vi "EnFlo_Hub.vi"() -> ()   [LabVIEW 2013]
uses:
  Anemometry Sub Vis/Controls/Launch_controls/Open_Calib.ctl
  Anemometry Sub Vis/Controls/Launch_controls/Open_Meas.ctl
  Anemometry Sub Vis/Controls/Launch_controls/Open_Enter_Temp.ctl
  Anemometry Sub Vis/Controls/Launch_controls/Multi_Run_Prog.ctl
  Anemometry Sub Vis/Controls/Launch_controls/EnFlo_arm.ctl
  Anemometry Sub Vis/Controls/Launch_controls/Fast_FID_Valve.ctl
  Anemometry Sub Vis/Controls/Launch_controls/Disp_Setup.ctl
  Anemometry Sub Vis/Controls/Launch_controls/EnFlo_Tun_Setup.ctl
  Anemometry Sub Vis/Controls/Launch_controls/User_Metadata.ctl
  Anemometry Sub Vis/Controls/Launch_controls/Trav_3D_move.ctl
  Anemometry Sub Vis/Controls/Launch_controls/Trav_Space.ctl
  Anemometry Sub Vis/Controls/Launch_controls/Tunnel_speed.ctl
  Anemometry Sub Vis/Controls/Launch_controls/Client_source_control.ctl
  Anemometry Sub Vis/Controls/Launch_controls/Hydrosonic_Manual.ctl
  Anemometry Sub Vis/Controls/Launch_controls/Preference_Panel.ctl
  Anemometry Sub Vis/Controls/Launch_controls/Hot_wire_Calculator.ctl
  Anemometry Sub Vis/Controls/Launch_controls/RW_X_Parker_Config.ctl
  Anemometry Sub Vis/Controls/Launch_controls/LDA_Alignment.ctl
  Anemometry Sub Vis/Controls/Launch_controls/Named_Serial_Comms.ctl
  Anemometry Sub Vis/Controls/Launch_controls/BSA_data_rates.ctl
  Anemometry Sub Vis/Controls/Launch_controls/Serial_Setup.ctl
  Anemometry Sub Vis/Controls/Launch_controls/Post_Process_icon.ctl
  Anemometry Sub Vis/Controls/Launch_controls/Edit_Ascii_file.ctl
  Anemometry Sub Vis/Controls/Launch_controls/Edit_Raw_DF.ctl
  Anemometry Sub Vis/Controls/Launch_controls/Results_file_plotter.ctl
  Anemometry Sub Vis/Controls/Launch_controls/Serial_Port_Names.ctl
  Anemometry Sub Vis/Controls/Launch_controls/Paul.ctl
  Anemometry Sub Vis/Controls/Launch_controls/Tom.ctl
  Anemometry Sub Vis/Controls/Launch_controls/Scani_Valve.ctl
  Anemometry Sub Vis/Controls/Launch_controls/Edit_sever_Channel.ctl
  Anemometry Sub Vis/Controls/Launch_controls/Day_file_plotter.ctl
  Anemometry Sub Vis/Controls/Launch_controls/Plot_Sever_Data.ctl
  Anemometry Sub Vis/Controls/Launch_controls/Adam_Table.ctl
  Anemometry Sub Vis/Controls/Launch_controls/Active_Channel_Control.ctl
  Anemometry Sub Vis/Controls/Setup.ctl
  Anemometry Sub Vis/Controls/Post_Process.ctl
  Anemometry Sub Vis/Controls/Preference_Mode.ctl
  Anemometry Sub Vis/Gen Trav/Trav_mode.ctl
  Anemometry Sub Vis/Controls/User_Specific_mode.ctl
  Anemometry Sub Vis/File/Setup_Filetype.ctl
  Anemometry Sub Vis/Calibration/Calib_mode.ctl
  Anemometry Sub Vis/Controls/Server_Comms.ctl
  Anemometry Sub Vis/Controls/App_Global.ctl
  Anemometry Sub Vis/Globals/Dynamic_call_global.ph.vi
  Anemometry Sub Vis/Globals/Constants_global.vi
  Anemometry Sub Vis/Globals/Preference_global.vi
  Anemometry Sub Vis/Globals/Meas_global.vi
  <vilib>/Platform/browser.llb/Open URL in Default Browser (string).vi
  Anemometry Sub Vis/Globals/Trav_pos_global.vi
  Anemometry Sub Vis/Acquisition/PWA/PWAtasksGLOBAL.vi
  Anemometry Sub Vis/Utilities/Email_transfer_global.vi
panel:
  out "List of ADAM channels to view":string[](array[string])
  out "List of ADAM control channels":string[](array[string])
  out "Analogue Dev Name":string="Dev2"
  out "Numeric":i32
  out "Rig Name":string="EnFlo Tunnel"
  out "All Users":path=path "/System Folder/Preferences/LabVIEW (EnFlo specific)/Meas Setups"
  out "Dummy Measurement":bool
  in  "stop":bool
  in  "Tab Control":T1(tab)
  in  "Tunnel Speed Control":T2
  in  "Traverse Space":T3
  in  "Trav 3D Move":T4 caption="3D Traverse Move"
  in  "User Metadata":T5
  in  "Multi Run Prog":T6
  in  "Enter Temp_Press":T7
  in  "Measurement Prog":T8 caption="Measurement"
  in  "Calibration Prog":T9 caption="Calibration"
  in  "Scani Valve":T10
  in  "LDA Alignment":T11
  in  "Hydrosonic Control":T12
  in  "Fast FID Valve":T13
  in  "Source Control":T14
  in  "Gas Release Setup":T15
  in  "EnFlo Tunnel Setup":T16
  in  "Heater Setup":bool caption="Inlet heater File"
  in  "EnFlo Arm":T17
  in  "EnFlo Tun Display":bool
  in  "Beam Check Positions":bool
  in  "Rig_Control":cluster{"Ch Name":string, "Boolean":bool}[](array[cluster])
  in  "ADAM Channels Control":T18 caption="Change Active Channels"
  in  "ADAM Scan Table":T19 caption="Run ADAM Scan Table"
  in  "Edit Server Channel":T20
  in  "Plot Server Channels":T21 caption="Plot Server Data"
  in  "Day Files Plotter":T22 caption="Plot Data From File"
  out "Current Values":cluster{"Ch Name":string, "Numeric":dbl}[](array[cluster])
  in  "Post_Pro_Results_Hierarchy":bool
  in  "Results File Plotter":T23
  in  "Edit Raw Data Files":T24
  in  "Edit ASCII File":T25
  in  "Post Process Raw Data":T26
  in  "Plot_FFID_Calibs.vi":bool
  in  "Top Level Traverse":bool
  in  "Show Manual Sync":bool
  in  "Sync to server now":bool
  in  "Port Names":T27
  in  "Serial Setup":T28
  in  "LDA Data Rate":T29
  in  "Named Serial Comms":T30
  in  "RW Trav Setup":T31
  in  "Hot Wire Calc":T32
  in  "Preference Panel":T33
  in  "Tom Lawton t.lawton@surrey.ac.uk":T34 caption="For hardware support"
  in  "Paul Hayden p.hayden@surrey.ac.uk":T35 caption="For software support"
  in  "Online Manual":bool
  out "VI Name":string
  out "Iterations":i32
  # "Or give us a call on Tel: 01483 689545"
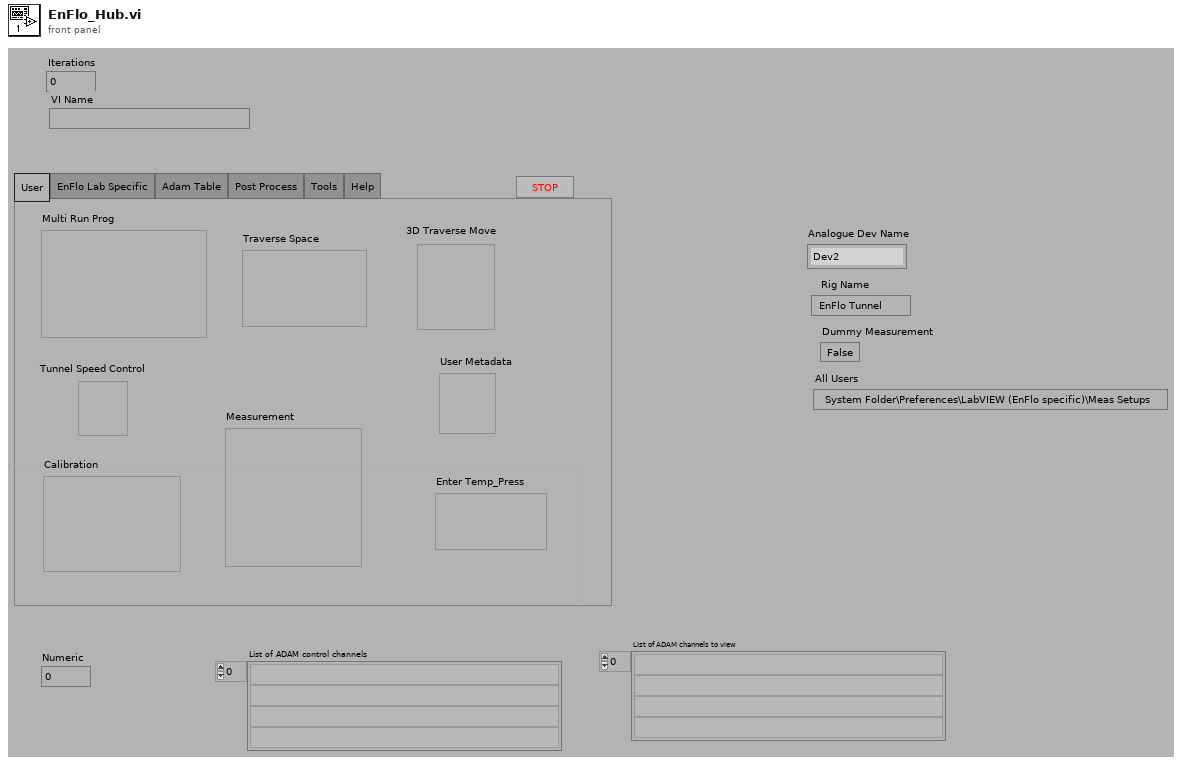
[diagram p1: front panel]
types:
  T1 = enum32{"User", "EnFlo Lab Specific", "Adam Table", "Post Process", "Tools", "Help"}
  T2 = typedef "Tunnel_speed.ctl" = bool
  T3 = typedef "Trav_Space.ctl" = bool
  T4 = typedef "Trav_3D_move.ctl" = bool
  T5 = typedef "User_Metadata.ctl" = bool
  T6 = typedef "Multi_Run_Prog.ctl" = bool
  T7 = typedef "Open_Enter_Temp.ctl" = bool
  T8 = typedef "Open_Meas.ctl" = bool
  T9 = typedef "Open_Calib.ctl" = bool
  T10 = typedef "Scani_Valve.ctl" = bool
  T11 = typedef "LDA_Alignment.ctl" = bool
  T12 = typedef "Hydrosonic_Manual.ctl" = bool
  T13 = typedef "Fast_FID_Valve.ctl" = bool
  T14 = typedef "Client_source_control.ctl" = bool
  T15 = typedef "Disp_Setup.ctl" = bool
  T16 = typedef "EnFlo_Tun_Setup.ctl" = bool
  T17 = typedef "EnFlo_arm.ctl" = bool
  T18 = typedef "Active_Channel_Control.ctl" = bool
  T19 = typedef "Adam_Table.ctl" = bool
  T20 = typedef "Edit_sever_Channel.ctl" = bool
  T21 = typedef "Plot_Sever_Data.ctl" = bool
  T22 = typedef "Day_file_plotter.ctl" = bool
  T23 = typedef "Results_file_plotter.ctl" = bool
  T24 = typedef "Edit_Raw_DF.ctl" = bool
  T25 = typedef "Edit_Ascii_file.ctl" = bool
  T26 = typedef "Post_Process_icon.ctl" = bool
  T27 = typedef "Serial_Port_Names.ctl" = bool
  T28 = typedef "Serial_Setup.ctl" = bool
  T29 = typedef "BSA_data_rates.ctl" = bool
  T30 = typedef "Named_Serial_Comms.ctl" = bool
  T31 = typedef "RW_X_Parker_Config.ctl" = bool
  T32 = typedef "Hot_wire_Calculator.ctl" = bool
  T33 = typedef "Preference_Panel.ctl" = bool
  T34 = typedef "Tom.ctl" = bool
  T35 = typedef "Paul.ctl" = bool
  T36 = typedef "Post_Process.ctl" = enum16{"Take New Data", "Post Process Raw Data File"}
  T37 = typedef "Setup.ctl" = enum16{"Run Program", "Show Setup", "Save Current Setup", "Setup Front Panel"}
  T38 = enum16{"Get Channel Names", "Get Current Value", "Update Channel Value", "Update Channel Description"}
  T39 = enum32{"Invalid", "Standard", "Closed", "Hidden", "Minimized", "Maximized"}
  T40 = enum32{"Bad", "Idle", "Run top level", "Running"}
  T41 = enum16{"Load From Excel File", "Save to Excel File"}
  T42 = typedef "Preference_Mode.ctl" = enum16{"Load Preferences from file", "Save Preferences to file", "Load, Edit then Save"}
  T43 = typedef "User_Specific_mode.ctl" = enum16{"Check VI only", "Run VI"}
  T44 = typedef "Trav_mode.ctl" = enum16{"Move traverse", "Read traverse position", "Teach Position"}
  T45 = typedef "Setup_Filetype.ctl" = enum16{"Measurement Setups", "Calibration Setups", "General", "Results File Plotter Setups", "Speed Calib Tweaks"}
  T46 = enum16{"Load Command File", "Save Command File", "Check Multi Run Prog", "Check Multi Run Prog With Live Moves", "Run Multi Run Prog"}
  T47 = typedef "Calib_mode.ctl" = enum16{"Show Setup", "Take a New Calibration Point", "Refit Curve", "Setup Front Panel"}
  T48 = typedef "Tunnel_Coordinates.ctl" = enum16{"Work in Tunnel Coordinates", "Work in Model Coordinates"}
  T49 = typedef "App_Global.ctl" = enum16{"Read Global", "Write to Global", "Initialise Array"}
  T50 = typedef "App_Ref_Cluster.ctl" = cluster{"Server IP & Port No":string, "Application reference":refnum<vi>}
  T51 = typedef "Server_Comms.ctl" = enum16{"Server Link Healthy", "Do Not Link To Server"}
  T52 = typedef "Ch_description_ADAM.ctl" = cluster{"Ch Name":string, "Type":T53, "Function":T54, "Ch State":T55, "Calibration type":T56, "A":dbl, "B":dbl, "C":dbl, "D":dbl, "Comments":string, "Address":T57, "String":string, "Duty":u16}
  T53 = typedef "Module_type_ADAM.ctl" = string
  T54 = typedef "Function_ADAM.ctl" = enum16{"Analogue Input", "Digital Input", "Event counter", "Event rate", "Analogue Output", "Digital Output", "Relay Output"}
  T55 = typedef "Channel_State.ctl" = enum16{"On", "Off", "Always On", "Always Off"}
  T56 = typedef "Calib_type_ADAM.ctl" = enum16{"Raw", "Bx + A", "Cx^2 + Bx + A", "Dx^3 + Cx^2 + Bx + A", "In Band", "Hi-Tec Q", "Hi-Tec M_dot", "Text"}
  T57 = typedef "Address.ctl" = cluster{"Main":i32, "Ch.":i32, "Sub":i32, "Port Name":string}
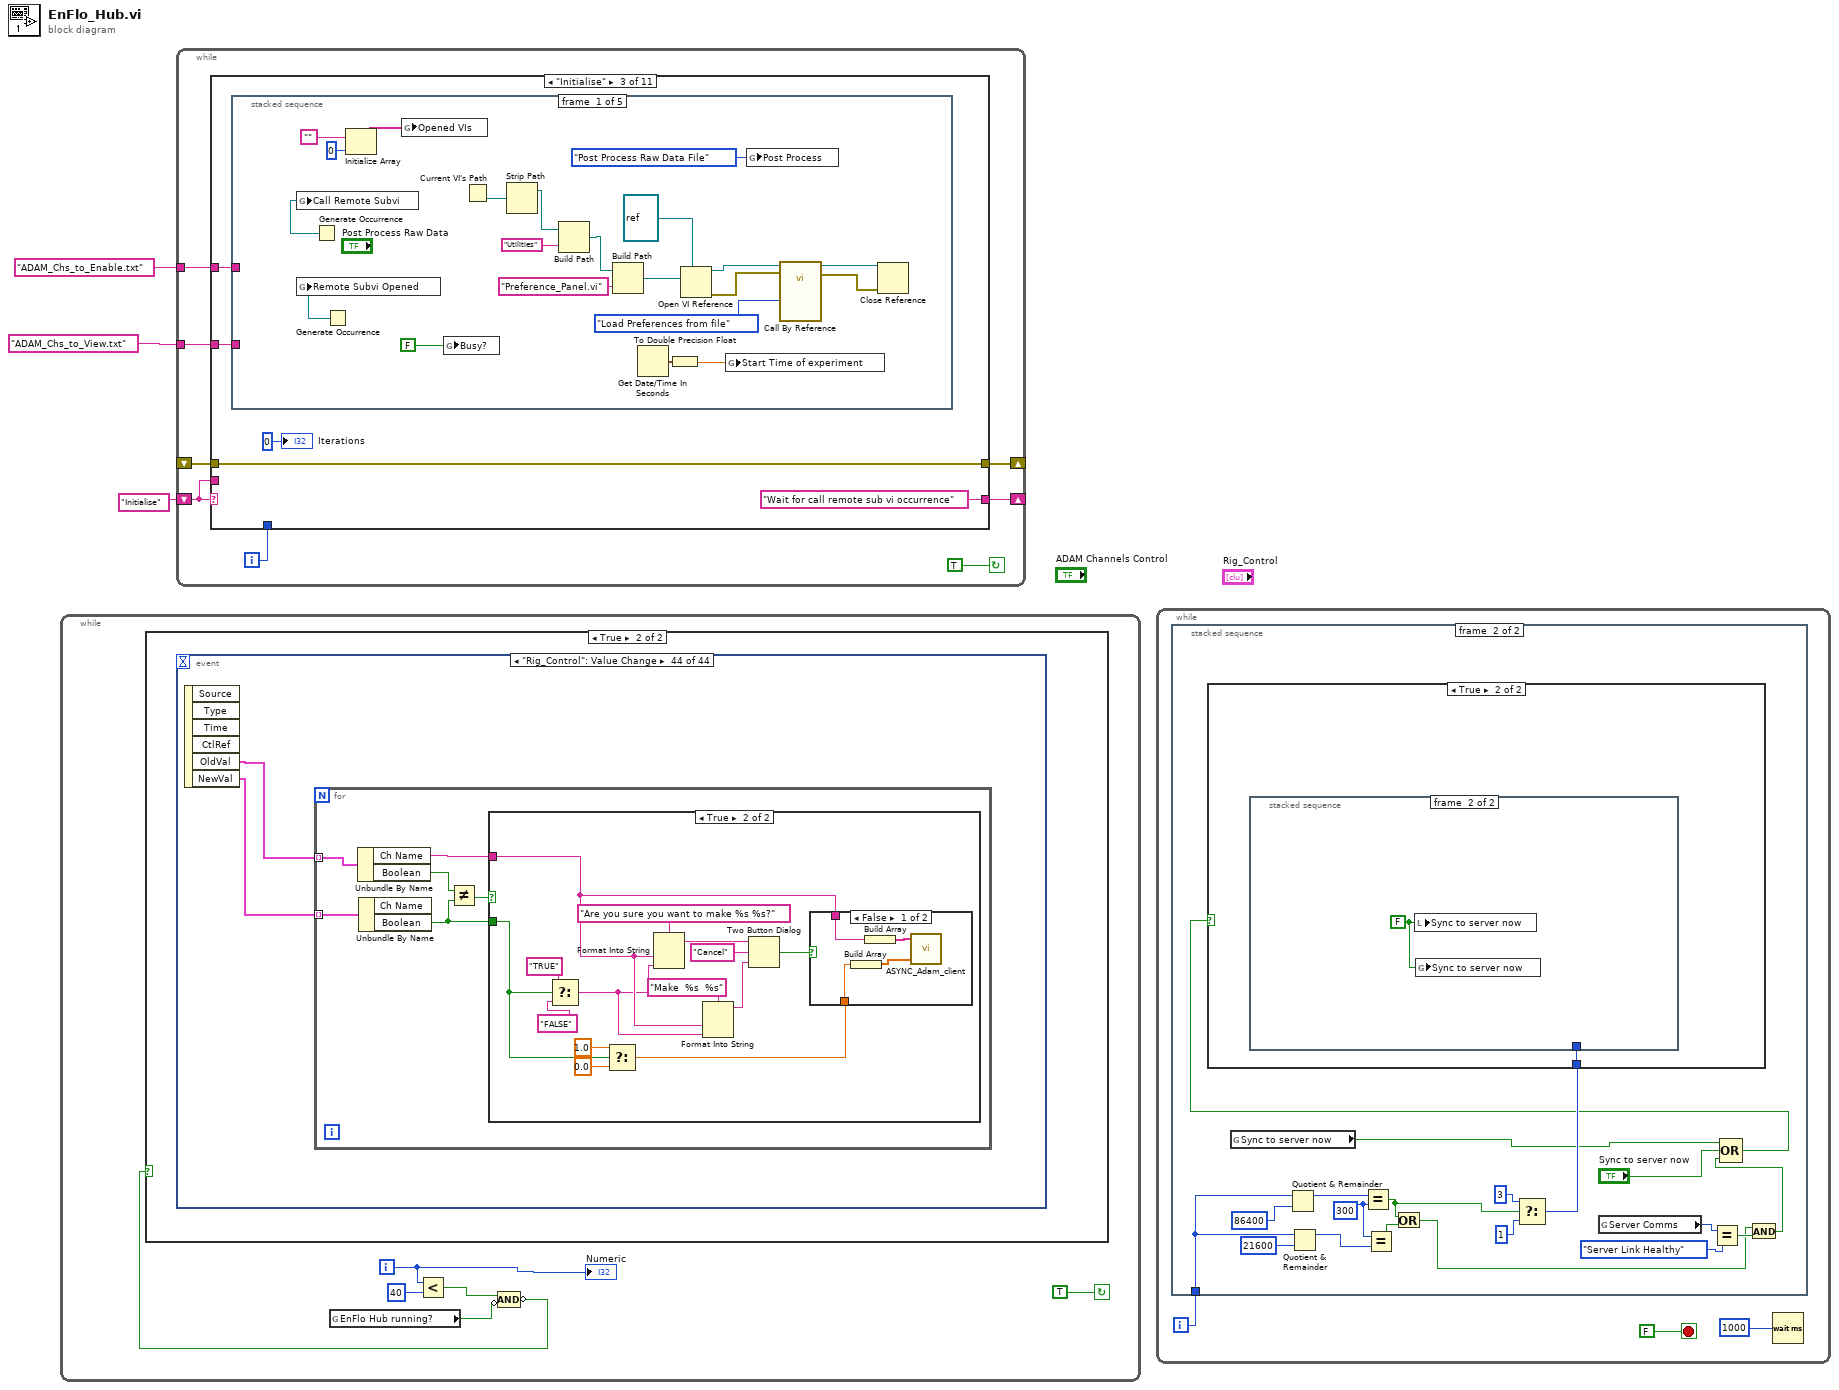
[diagram p0: block diagram]
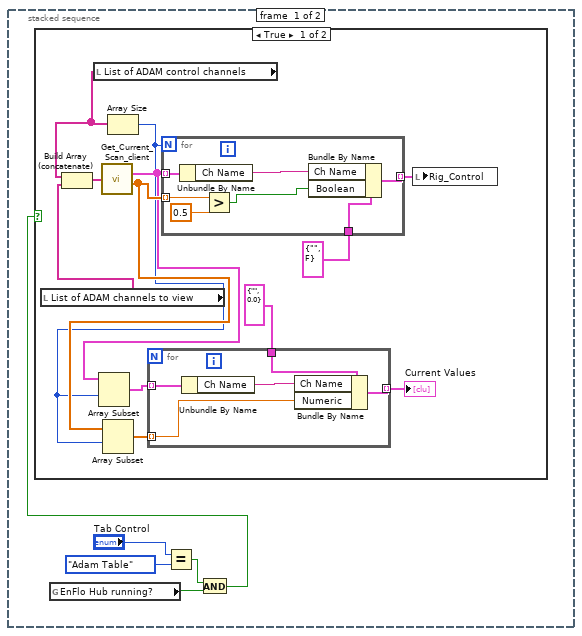
[diagram p2: hidden frame]
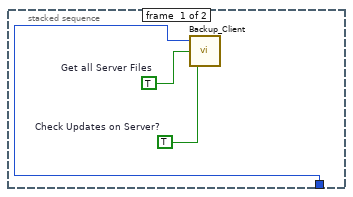
[diagram p5: hidden frame]
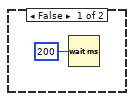
[diagram p6: hidden frame]
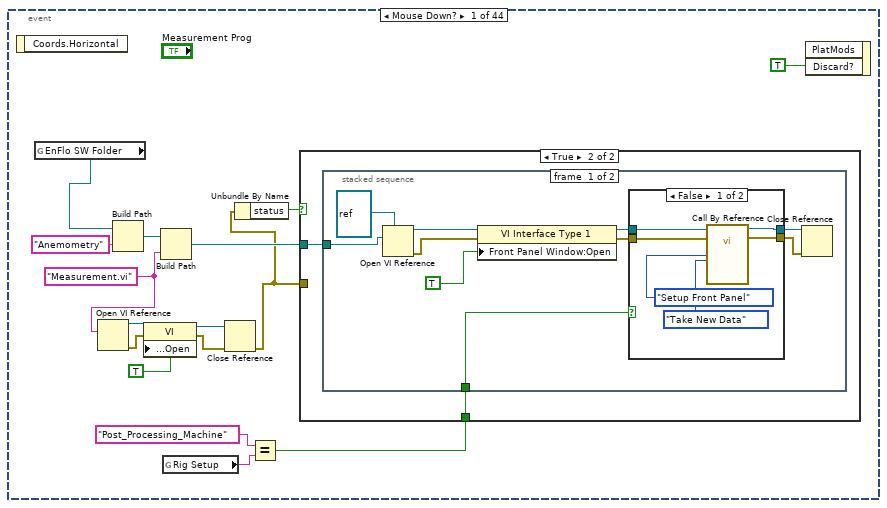
[diagram p7: hidden frame]
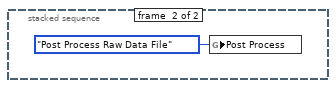
[diagram p10: hidden frame]
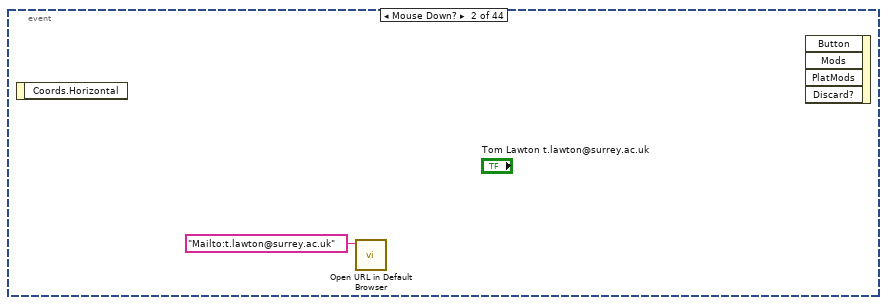
[diagram p11: hidden frame]
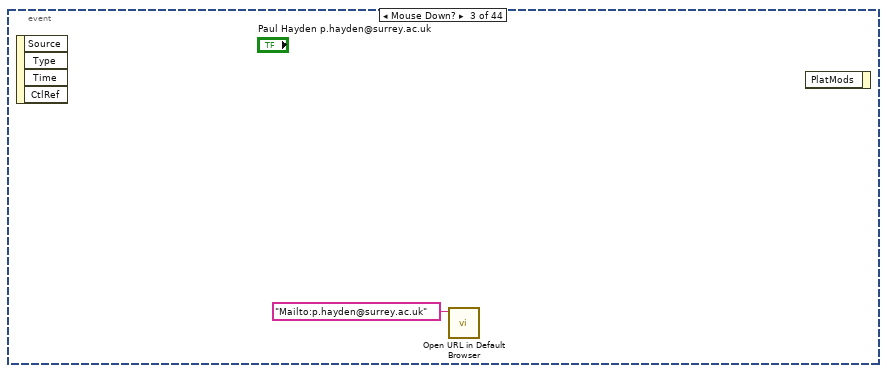
[diagram p12: hidden frame]
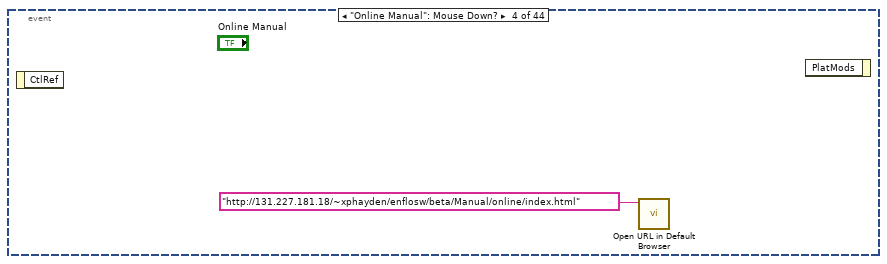
[diagram p13: hidden frame]
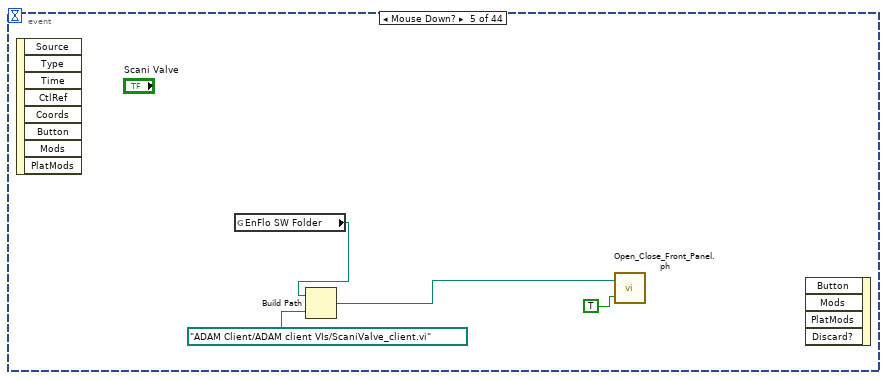
[diagram p14: hidden frame]
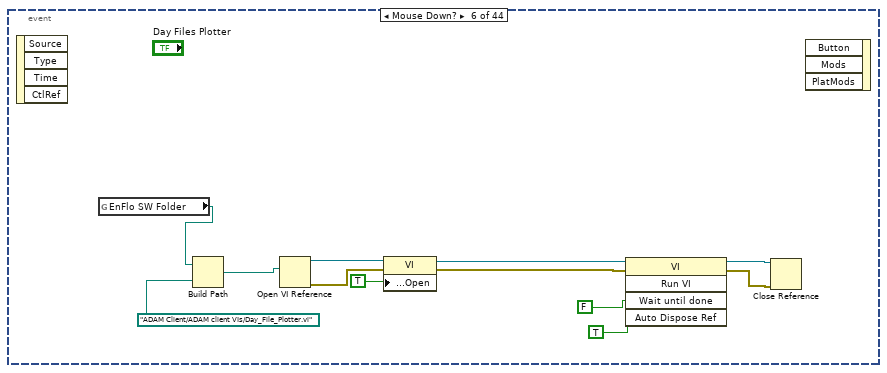
[diagram p15: hidden frame]
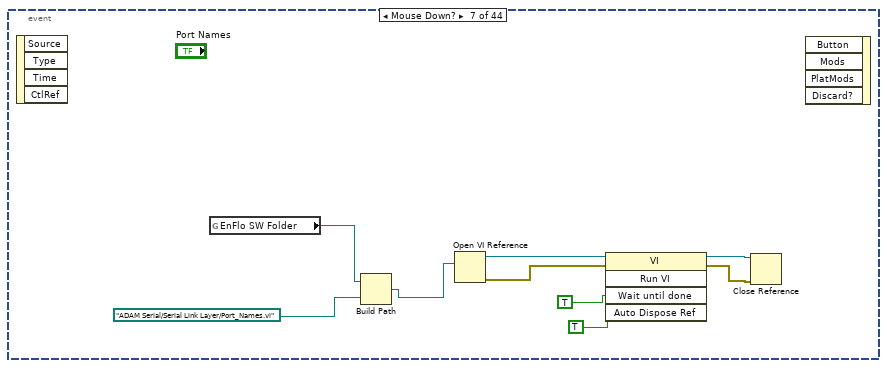
[diagram p16: hidden frame]
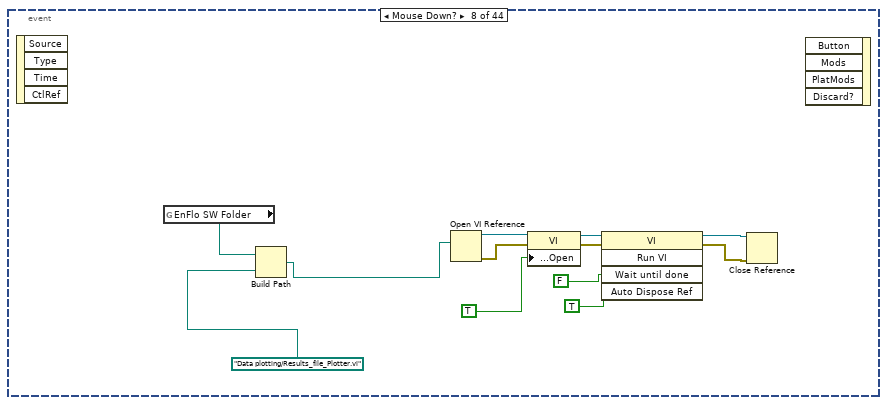
[diagram p17: hidden frame]
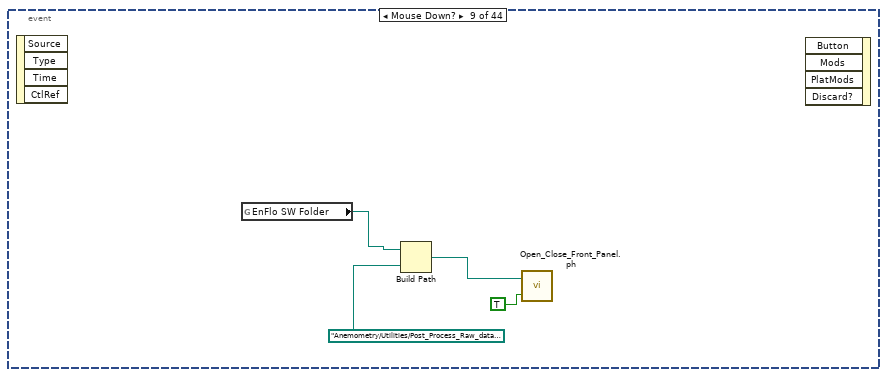
[diagram p18: hidden frame]
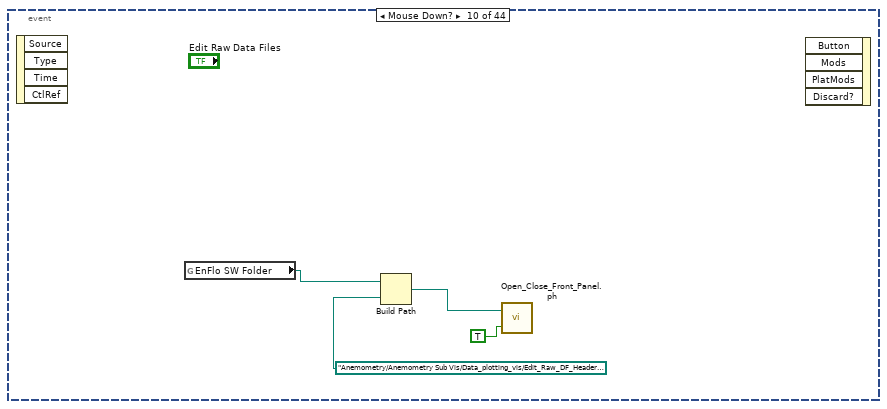
[diagram p19: hidden frame]
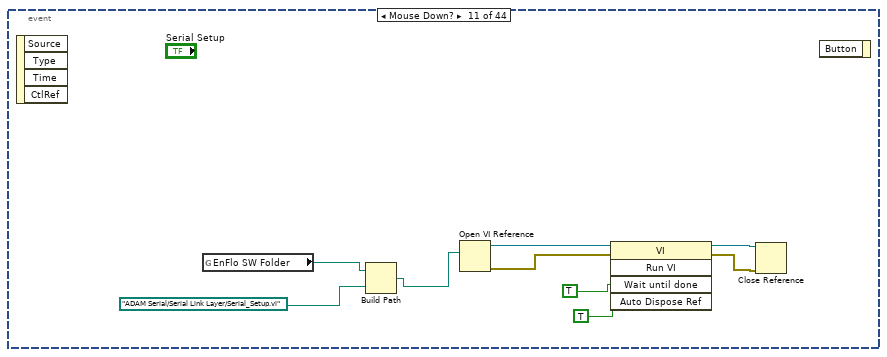
[diagram p20: hidden frame]
diagram:
  n1 = while {
    i -> [w8]
    stop <- TRUE continue-if-true
    n2 = global read "Dynamic_call_global.ph.vi" "EnFlo Hub running?"() -> (w6:bool)
    n3 = Less?(x=w8, y=40) -> (x < y?=w5:bool)
    n4 = Compound Arithmetic op=AND(w5, invert w6) -> (invert w4:bool)
    n5 = case shown="True" w4 {
      frame False {
        n6 = Wait (ms)(milliseconds to wait=u32 200) -> ()  [unwired: 1 out]
      }
      frame True {
        n7 = event shown="[43] \"Rig_Control\": Value Change" {
          selector: _ -> [_ _ _ _ _ _ _ _ _ _ _ _ _ _ _ _ _ _ _ _ _ _ _ _ _ _ _ _ _ _ _ _ _ _ _ _ _ _ _ _ _ _ _ _]
          dyn-events: _ -> [_ _ _ _ _ _ _ _ _ _ _ _ _ _ _ _ _ _ _ _ _ _ _ _ _ _ _ _ _ _ _ _ _ _ _ _ _ _ _ _ _ _ _ _]
          timeout: _ -> [_ _ _ _ _ _ _ _ _ _ _ _ _ _ _ _ _ _ _ _ _ _ _ _ _ _ _ _ _ _ _ _ _ _ _ _ _ _ _ _ _ _ _ _]
          event Mouse Down? {
            w19 = "Measurement.vi" ("name or relative path")
            n8 = event-data() -> ()  [unwired: 2 out]
            n9 = global read "Constants_global.vi" "EnFlo SW Folder"() -> (w22:path)
            n10 = Open VI Reference(vi path=w19) -> (vi reference=w18:refnum<vi>, error out=w17:errorcluster)  [unwired: 1 in, 4 out]
            n11 = Build Path(base path=w22, name or relative path="Anemometry") -> (appended path=w25:path)
            n12 = property class="VI"(reference=w18, error in=w17, "Front Panel Window:Open"=TRUE) -> (reference out=w15:refnum<vi>, error out=w16:errorcluster)
            n13 = Build Path(base path=w25, name or relative path=w19) -> (appended path=w23:path)
            n14 = global read "Preference_global.vi" "Rig Setup"() -> (w13:string)
            n15 = Close Reference(reference=w15, error in (no error)=w16) -> (error out=w14:errorcluster)
            n16 = Unbundle By Name(w14) -> ("status"=w24:bool)
            n17 = Equal?(x="Post_Processing_Machine" ("Rig Setup"), y=w13) -> (x = y?=w11:bool)
            n18 = case shown="True" w24 {
              tunnel: w23 -> [_ w28]
              tunnel: w14 -> [_ _]
              tunnel: w11 -> [_ w27]
              frame False {
              }
              frame True {
                n19 = stacked-sequence {
                  tunnel: w28 -> [w38 _]
                  tunnel: w27 -> [w29 _]
                  frame #0 {
                    n20 = Open VI Reference(type specifier VI Refnum (for type only)=refnum<vi> refnum, vi path=w38) -> (vi reference=w36:refnum<vi>, error out=w35:errorcluster)  [unwired: 1 in, 3 out]
                    n21 = property class="VI Interface Type 1"(reference=w36, error in=w35, "Front Panel Window:Open"=TRUE) -> (reference out=w31:refnum<vi>, error out=w30:errorcluster)
                    n22 = case shown="False" w29 {
                      tunnel: [w44 w46] -> w34
                      tunnel: [w43 w45] -> w33
                      tunnel: w31 -> [w42 w46]
                      tunnel: w30 -> [w41 w45]
                      frame False {
                        n23 = call-by-ref "?"(reference=w42, error in=w41, "setup"=Setup."Setup Front Panel", "Post Process"=Post_Process."Take New Data") -> (reference out=w44:refnum<vi>, error out=w43:errorcluster)  [unwired: 16 in, 2 out]
                      }
                      frame True {
                      }
                    }
                    n24 = Close Reference(reference=w34, error in (no error)=w33) -> ()  [unwired: 1 out]
                  }
                  frame #1 {
                    n25 = global write "Meas_global.vi" "Post Process"(Post_Process."Post Process Raw Data File" ("Post Process")) -> ()
                  }
                }
              }
            }
            n26 = event-data("Discard?"=TRUE) -> ()  [unwired: 1 in, 2 out]
          }
          event Mouse Down? {
            n27 = event-data() -> ()  [unwired: 2 out]
            n28 = call-poly <vilib>:"Open URL in Default Browser.vi"("URL"="Mailto:t.lawton@surrey.ac.uk") -> ()  [unwired: 1 in, 6 out]
            n29 = event-data() -> ()  [unwired: 1 in, 5 out]
          }
          event Mouse Down? {
            n30 = event-data() -> ()  [unwired: 5 out]
            n31 = call-poly <vilib>:"Open URL in Default Browser.vi"("URL"="Mailto:p.hayden@surrey.ac.uk") -> ()  [unwired: 1 in, 6 out]
            n32 = event-data() -> ()  [unwired: 1 in, 2 out]
          }
          event "Online Manual": Mouse Down? {
            n33 = event-data() -> ()  [unwired: 2 out]
            n34 = call-poly <vilib>:"Open URL in Default Browser.vi"("URL"="http://131.227.181.18/~xphayden/enflosw/beta/Manual/online/index.html") -> ()  [unwired: 1 in, 6 out]
            n35 = event-data() -> ()  [unwired: 1 in, 2 out]
          }
          event Mouse Down? {
            n36 = event-data() -> ()  [unwired: 9 out]
            n37 = global read "Constants_global.vi" "EnFlo SW Folder"() -> (w51:path)
            n38 = Build Path(base path=w51, name or relative path=path "ADAM Client/ADAM client VIs/ScaniValve_client.vi") -> (appended path=w54:path)
            n39 = call "Open_Close_Front_Panel.ph.vi"("Front Panel Window:Open"=TRUE, "VI path"=w54) -> ()  [unwired: 2 out]
            n40 = event-data() -> ()  [unwired: 1 in, 5 out]
          }
          event Mouse Down? {
            n41 = event-data() -> ()  [unwired: 5 out]
            n42 = global read "Constants_global.vi" "EnFlo SW Folder"() -> (w55:path)
            n43 = Build Path(base path=w55, name or relative path=path "ADAM Client/ADAM client VIs/Day_File_Plotter.vi") -> (appended path=w61:path)
            n44 = Open VI Reference(vi path=w61) -> (vi reference=w62:refnum<vi>, error out=w64:errorcluster)  [unwired: 2 in, 3 out]
            n45 = property class="VI"(reference=w62, error in=w64, "Front Panel Window:Open"=TRUE) -> (reference out=w66:refnum<vi>, error out=w65:errorcluster)
            n46 = invoke class="VI" method="Run VI"(reference=w66, error in=w65, "Wait until done"=FALSE, "Auto Dispose Ref"=TRUE) -> (reference out=w57:refnum<vi>, error out=w58:errorcluster)  [unwired: 1 in, 3 out]
            n47 = Close Reference(reference=w57, error in (no error)=w58) -> ()  [unwired: 1 out]
            n48 = event-data() -> ()  [unwired: 1 in, 4 out]
          }
          event Mouse Down? {
            n49 = event-data() -> ()  [unwired: 5 out]
            n50 = global read "Constants_global.vi" "EnFlo SW Folder"() -> (w67:path)
            n51 = Build Path(base path=w67, name or relative path=path "ADAM Serial/Serial Link Layer/Port_Names.vi") -> (appended path=w69:path)
            n52 = Open VI Reference(vi path=w69) -> (vi reference=w74:refnum<vi>, error out=w75:errorcluster)  [unwired: 1 in, 4 out]
            n53 = invoke class="VI" method="Run VI"(reference=w74, error in=w75, "Wait until done"=TRUE, "Auto Dispose Ref"=TRUE) -> (reference out=w70:refnum<vi>, error out=w71:errorcluster)  [unwired: 1 in, 3 out]
            n54 = Close Reference(reference=w70, error in (no error)=w71) -> ()  [unwired: 1 out]
            n55 = event-data() -> ()  [unwired: 1 in, 5 out]
          }
          event Mouse Down? {
            n56 = event-data() -> ()  [unwired: 5 out]
            n57 = global read "Constants_global.vi" "EnFlo SW Folder"() -> (w76:path)
            n58 = Build Path(base path=w76, name or relative path=path "Data plotting/Results_file_Plotter.vi") -> (appended path=w79:path)
            n59 = Open VI Reference(vi path=w79) -> (vi reference=w81:refnum<vi>, error out=w78:errorcluster)  [unwired: 1 in, 4 out]
            n60 = property class="VI"(reference=w81, error in=w78, "Front Panel Window:Open"=TRUE) -> (reference out=w82:refnum<vi>, error out=w83:errorcluster)
            n61 = invoke class="VI" method="Run VI"(reference=w82, error in=w83, "Wait until done"=FALSE, "Auto Dispose Ref"=TRUE) -> (reference out=w84:refnum<vi>, error out=w85:errorcluster)  [unwired: 1 in, 3 out]
            n62 = Close Reference(reference=w84, error in (no error)=w85) -> ()  [unwired: 1 out]
            n63 = event-data() -> ()  [unwired: 1 in, 5 out]
          }
          event Mouse Down? {
            n64 = event-data() -> ()  [unwired: 5 out]
            n65 = global read "Constants_global.vi" "EnFlo SW Folder"() -> (w88:path)
            n66 = Build Path(base path=w88, name or relative path=path "Anemometry/Utilities/Post_Process_Raw_data.vi") -> (appended path=w90:path)
            n67 = call "Open_Close_Front_Panel.ph.vi"("Front Panel Window:Open"=TRUE, "VI path"=w90) -> ()  [unwired: 2 out]
            n68 = event-data() -> ()  [unwired: 1 in, 5 out]
          }
          event Mouse Down? {
            n69 = event-data() -> ()  [unwired: 5 out]
            n70 = global read "Constants_global.vi" "EnFlo SW Folder"() -> (w92:path)
            n71 = Build Path(base path=w92, name or relative path=path "Anemometry/Anemometry Sub Vis/Data_plotting_vis/Edit_Raw_DF_Header.vi") -> (appended path=w94:path)
            n72 = call "Open_Close_Front_Panel.ph.vi"("Front Panel Window:Open"=TRUE, "VI path"=w94) -> ()  [unwired: 2 out]
            n73 = event-data() -> ()  [unwired: 1 in, 5 out]
          }
          event Mouse Down? {
            n74 = event-data() -> ()  [unwired: 5 out]
            n75 = global read "Constants_global.vi" "EnFlo SW Folder"() -> (w96:path)
            n76 = Build Path(base path=w96, name or relative path=path "ADAM Serial/Serial Link Layer/Serial_Setup.vi") -> (appended path=w98:path)
            n77 = Open VI Reference(vi path=w98) -> (vi reference=w103:refnum<vi>, error out=w104:errorcluster)  [unwired: 1 in, 4 out]
            n78 = invoke class="VI" method="Run VI"(reference=w103, error in=w104, "Wait until done"=TRUE, "Auto Dispose Ref"=TRUE) -> (reference out=w99:refnum<vi>, error out=w100:errorcluster)  [unwired: 1 in, 3 out]
            n79 = Close Reference(reference=w99, error in (no error)=w100) -> ()  [unwired: 1 out]
            n80 = event-data() -> ()  [unwired: 1 in, 2 out]
          }
          event Mouse Down? {
            n81 = event-data() -> ()  [unwired: 5 out]
            n82 = global read "Constants_global.vi" "EnFlo SW Folder"() -> (w106:path)
            n83 = Build Path(base path=w106, name or relative path=path "ADAM Serial/Serial Link Layer/Named_Serial_Comms.vi") -> (appended path=w108:path)
            n84 = call "Open_Close_Front_Panel.ph.vi"("Front Panel Window:Open"=TRUE, "VI path"=w108) -> ()  [unwired: 2 out]
            n85 = event-data() -> ()  [unwired: 1 in, 5 out]
          }
          event Mouse Down? {
            n86 = event-data() -> ()  [unwired: 5 out]
            n87 = global read "Constants_global.vi" "EnFlo SW Folder"() -> (w109:path)
            n88 = Build Path(base path=w109, name or relative path=path "Anemometry/Anemometry Sub Vis/LDA/LDA_data_rate.vi") -> (appended path=w111:path)
            n89 = call "Open_Close_Front_Panel.ph.vi"("Front Panel Window:Open"=TRUE, "VI path"=w111) -> ()  [unwired: 2 out]
            n90 = event-data() -> ()  [unwired: 1 in, 2 out]
          }
          event Mouse Down? {
            n91 = event-data() -> ()  [unwired: 5 out]
            n92 = global read "Constants_global.vi" "EnFlo SW Folder"() -> (w123:path)
            n93 = Build Path(base path=w123, name or relative path=path "ADAM Client/ADAM client VIs/Control_Channel_Status.vi") -> (appended path=w113:path)
            n94 = Open VI Reference(vi path=w113) -> (vi reference=w116:refnum<vi>, error out=w114:errorcluster)  [unwired: 1 in, 4 out]
            n95 = property class="VI"(reference=w116, error in=w114, "Front Panel Window:Open"=TRUE) -> (reference out=w117:refnum<vi>, error out=w118:errorcluster)
            n96 = invoke class="VI" method="Run VI"(reference=w117, error in=w118, "Wait until done"=FALSE, "Auto Dispose Ref"=TRUE) -> (reference out=w119:refnum<vi>, error out=w120:errorcluster)  [unwired: 1 in, 3 out]
            n97 = Close Reference(reference=w119, error in (no error)=w120) -> ()  [unwired: 1 out]
            n98 = event-data() -> ()  [unwired: 1 in, 2 out]
          }
          event Mouse Down? {
            n99 = event-data() -> ()  [unwired: 5 out]
            n100 = global read "Constants_global.vi" "EnFlo SW Folder"() -> (w125:path)
            n101 = Build Path(base path=w125, name or relative path=path "Anemometry/Utilities/LDA_Beam_Alignment.vi") -> (appended path=w127:path)
            n102 = call "Open_Close_Front_Panel.ph.vi"("Front Panel Window:Open"=TRUE, "VI path"=w127) -> ()  [unwired: 2 out]
            n103 = event-data() -> ()  [unwired: 1 in, 5 out]
          }
          event Mouse Down? {
            w130 = FALSE  # Wait until done
            n104 = event-data() -> ()  [unwired: 5 out]
            n105 = call "Run_Enter_Temp.vi"("Wait until done"=w130) -> ()  [unwired: 1 out]
            n106 = event-data("Discard?"=TRUE) -> ()  [unwired: 1 in, 4 out]
          }
          event Mouse Down? {
            n107 = event-data() -> ()  [unwired: 5 out]
            n108 = global read "Constants_global.vi" "EnFlo SW Folder"() -> (w131:path)
            n109 = Build Path(base path=w131, name or relative path=path "Anemometry/Utilities/Edit_ASCI_file.vi") -> (appended path=w134:path)
            n110 = call "Open_Close_Front_Panel.ph.vi"("Front Panel Window:Open"=TRUE, "VI path"=w134) -> ()  [unwired: 2 out]
            n111 = event-data() -> ()  [unwired: 1 in, 5 out]
          }
          event "Heater Setup": Mouse Down? {
            n112 = event-data() -> ()  [unwired: 5 out]
            n113 = global read "Constants_global.vi" "EnFlo SW Folder"() -> (w135:path)
            n114 = Build Path(base path=w135, name or relative path=path "Anemometry/Utilities/Create_Heater_Setpoints_File.vi") -> (appended path=w138:path)
            n115 = call "Open_Close_Front_Panel.ph.vi"("Front Panel Window:Open"=TRUE, "VI path"=w138) -> ()  [unwired: 2 out]
            n116 = event-data() -> ()  [unwired: 1 in, 5 out]
          }
          event Mouse Down? {
            n117 = event-data() -> ()  [unwired: 5 out]
            n118 = global read "Constants_global.vi" "EnFlo SW Folder"() -> (w139:path)
            n119 = Build Path(base path=w139, name or relative path=path "ADAM Client/Sub VIs/Gas_Release_Control.vi") -> (appended path=w142:path)
            n120 = call "Open_Close_Front_Panel.ph.vi"("Front Panel Window:Open"=TRUE, "VI path"=w142) -> ()  [unwired: 2 out]
            n121 = event-data() -> ()  [unwired: 1 in, 5 out]
          }
          event Mouse Down? {
            n122 = event-data() -> ()  [unwired: 5 out]
            n123 = global read "Constants_global.vi" "EnFlo SW Folder"() -> (w143:path)
            n124 = Build Path(base path=w143, name or relative path=path "ADAM Client/ADAM client VIs/Edit_Server_Channel.vi") -> (appended path=w153:path)
            n125 = Open VI Reference(type specifier VI Refnum (for type only)=refnum<vi> refnum, vi path=w153) -> (vi reference=w146:refnum<vi>, error out=w147:errorcluster)  [unwired: 1 in, 3 out]
            n126 = property class="VI Interface Type 2"(reference=w146, error in=w147, "Front Panel Window:Open"=TRUE) -> (reference out=w149:refnum<vi>, error out=w150:errorcluster)
            n127 = call-by-ref "?"(reference=w149, error in=w150, "Mode"=T38."Get Channel Names") -> (reference out=w151:refnum<vi>, error out=w152:errorcluster)  [unwired: 5 in]
            n128 = Close Reference(reference=w151, error in (no error)=w152) -> ()  [unwired: 1 out]
            n129 = event-data() -> ()  [unwired: 1 in, 5 out]
          }
          event "EnFlo Tun Display": Mouse Down? {
            n130 = event-data() -> ()  [unwired: 9 out]
            n131 = global read "Constants_global.vi" "EnFlo SW Folder"() -> (w166:path)
            n132 = Build Path(base path=w166, name or relative path=path "Anemometry/Utilities/EnFlo_Tunnel_Display.vi") -> (appended path=w161:path)
            n133 = Open VI Reference(vi path=w161) -> (vi reference=w160:refnum<vi>, error out=w159:errorcluster)  [unwired: 5 in]
            n134 = invoke class="VI" method="FP.Open"(reference=w160, error in=w159, "Activate"=TRUE ("Activate?"), "State"=T39."Standard") -> (reference out=w158:refnum<vi>, error out=w157:errorcluster)  [unwired: 1 in, 3 out]
            n135 = invoke class="VI" method="Run VI"(reference=w158, error in=w157, "Wait until done"=FALSE ("Wait Until Done"), "Auto Dispose Ref"=FALSE ("Wait until done")) -> (reference out=w162:refnum<vi>, error out=w163:errorcluster)  [unwired: 1 in, 3 out]
            n136 = Close Reference(reference=w162, error in (no error)=w163) -> ()  [unwired: 1 out]
            n137 = event-data() -> ()  [unwired: 5 in, 1 out]
          }
          event Mouse Down? {
            n138 = event-data() -> ()  [unwired: 5 out]
            n139 = global read "Constants_global.vi" "EnFlo SW Folder"() -> (w168:path)
            n140 = Build Path(base path=w168, name or relative path=path "ADAM Client/ADAM client VIs/Set_Tunnel_Speed.vi") -> (appended path=w171:path)
            n141 = call "Open_Close_Front_Panel.ph.vi"("Front Panel Window:Open"=TRUE, "VI path"=w171) -> ()  [unwired: 2 out]
            n142 = event-data() -> ()  [unwired: 1 in, 5 out]
          }
          event Mouse Down? {
            n143 = event-data() -> ()  [unwired: 5 out]
            n144 = global read "Constants_global.vi" "EnFlo SW Folder"() -> (w172:path)
            n145 = Build Path(base path=w172, name or relative path=path "ADAM Client/ADAM client VIs/Plot_Server_Data.vi") -> (appended path=w175:path)
            n146 = Open VI Reference(vi path=w175) -> (vi reference=w177:refnum<vi>, error out=w174:errorcluster)  [unwired: 1 in, 4 out]
            n147 = property class="VI"(reference=w177, error in=w174, "Front Panel Window:Open"=TRUE) -> (reference out=w178:refnum<vi>, error out=w179:errorcluster)
            n148 = invoke class="VI" method="Run VI"(reference=w178, error in=w179, "Wait until done"=FALSE, "Auto Dispose Ref"=TRUE) -> (reference out=w180:refnum<vi>, error out=w181:errorcluster)  [unwired: 1 in, 3 out]
            n149 = Close Reference(reference=w180, error in (no error)=w181) -> ()  [unwired: 1 out]
            n150 = event-data() -> ()  [unwired: 1 in, 5 out]
          }
          event Mouse Down? {
            n151 = event-data() -> ()  [unwired: 5 out]
            n152 = global read "Constants_global.vi" "EnFlo SW Folder"() -> (w191:path)
            n153 = Build Path(base path=w191, name or relative path=path "ADAM Server/ADAM_scan_table.vi") -> (appended path=w189:path)
            n154 = Open VI Reference(vi path=w189) -> (vi reference=w192:refnum<vi>, error out=w193:errorcluster)  [unwired: 1 in, 4 out]
            n155 = property class="VI"(reference=w192, error in=w193) -> (reference out=w187:refnum<vi>, error out=w186:errorcluster, "Execution:State"=w194:T40)
            n156 = Equal?(x=w194, y=T40."Run top level" ("Execution:State")) -> (x = y?=w188:bool)
            n157 = case shown="False" w188 {
              tunnel: w187 -> [w199 w216]
              tunnel: w186 -> [w198 w215]
              tunnel: [w197 w216] -> w185
              tunnel: [w196 w215] -> w184
              frame False {
                n158 = Two Button Dialog(message="Are you sure that you want to Run the ADAM Scan table on this machine?", 1:"Run" ("F button name (\"Cancel\")"), 2:"Cancel" ("T button name (\"OK\")")) -> (T button?=w200:bool)
                n159 = case shown="False" w200 {
                  tunnel: w199 -> [w207 w214]
                  tunnel: w198 -> [w206 w213]
                  tunnel: [w205 w214] -> w197
                  tunnel: [w204 w213] -> w196
                  frame False {
                    n160 = property class="VI"(reference=w207, error in=w206, "Front Panel Window:Open"=TRUE) -> (reference out=w211:refnum<vi>, error out=w210:errorcluster)
                    n161 = invoke class="VI" method="Run VI"(reference=w211, error in=w210, "Wait until done"=FALSE, "Auto Dispose Ref"=TRUE) -> (reference out=w205:refnum<vi>, error out=w204:errorcluster)  [unwired: 1 in, 3 out]
                  }
                  frame True {
                  }
                }
              }
              frame True {
              }
            }
            n162 = event-data() -> ()  [unwired: 1 in, 2 out]
            n163 = Close Reference(reference=w185, error in (no error)=w184) -> ()  [unwired: 1 out]
          }
          event Mouse Down? {
            n164 = event-data() -> ()  [unwired: 5 out]
            n165 = global read "Constants_global.vi" "EnFlo SW Folder"() -> (w219:path)
            n166 = Build Path(base path=w219, name or relative path=path "ADAM Serial/Instrument drivers/Traverses/~subVIs/Read_Write_Trav_Config.vi") -> (appended path=w220:path)
            n167 = Build Path(base path=w219, name or relative path=path "ADAM Serial/Instrument drivers/Traverses/~subVIs/DriveConfigGlobal.vi") -> (appended path=w221:path)
            n168 = flat-sequence {
              tunnel: w221 -> [w222]
              tunnel: w220 -> [w224]
              frame #0 {
                n169 = call "Open_Close_Front_Panel.ph.vi"("Front Panel Window:Open"=TRUE, "VI path"=w222) -> ()  [unwired: 2 out]
              }
              frame #1 {
                n170 = call "Open_Close_Front_Panel.ph.vi"("Front Panel Window:Open"=TRUE, "VI path"=w224) -> ()  [unwired: 2 out]
              }
            }
            n171 = event-data() -> ()  [unwired: 1 in, 5 out]
          }
          event Mouse Down? {
            n172 = event-data() -> ()  [unwired: 5 out]
            n173 = global read "Constants_global.vi" "EnFlo SW Folder"() -> (w226:path)
            n174 = Build Path(base path=w226, name or relative path=path "Anemometry/Utilities/Hot_wire_Calculator.vi") -> (appended path=w229:path)
            n175 = call "Open_Close_Front_Panel.ph.vi"("Front Panel Window:Open"=TRUE, "VI path"=w229) -> ()  [unwired: 2 out]
            n176 = event-data() -> ()  [unwired: 1 in, 5 out]
          }
          event "Show Manual Sync": Mouse Down {
            n177 = event-data() -> ()  [unwired: 9 out]
            n178 = global read "Constants_global.vi" "EnFlo SW Folder"() -> (w230:path)
            n179 = Build Path(base path=w230, name or relative path=path "Anemometry/Utilities/EnFlo_Data_Sync_Manual.vi") -> (appended path=w233:path)
            n180 = call "Open_Close_Front_Panel.ph.vi"("Front Panel Window:Open"=TRUE, "VI path"=w233) -> ()  [unwired: 2 out]
          }
          event "Plot_FFID_Calibs.vi": Mouse Down {
            n181 = event-data() -> ()  [unwired: 9 out]
            n182 = global read "Constants_global.vi" "EnFlo SW Folder"() -> (w244:path)
            n183 = Build Path(base path=w244, name or relative path=path "ADAM Client/ADAM client VIs/Plot_FFID_Calibs.vi") -> (appended path=w234:path)
            n184 = Open VI Reference(vi path=w234) -> (vi reference=w237:refnum<vi>, error out=w235:errorcluster)  [unwired: 1 in, 4 out]
            n185 = property class="VI"(reference=w237, error in=w235, "Front Panel Window:Open"=TRUE) -> (reference out=w238:refnum<vi>, error out=w239:errorcluster)
            n186 = invoke class="VI" method="Run VI"(reference=w238, error in=w239, "Wait until done"=FALSE, "Auto Dispose Ref"=TRUE) -> (reference out=w240:refnum<vi>, error out=w241:errorcluster)  [unwired: 1 in, 3 out]
            n187 = Close Reference(reference=w240, error in (no error)=w241) -> ()  [unwired: 1 out]
          }
          event "Beam Check Positions": Mouse Down {
            n188 = event-data() -> ()  [unwired: 9 out]
            n189 = global read "Constants_global.vi" "EnFlo SW Folder"() -> (w256:path)
            n190 = Build Path(base path=w256, name or relative path=path "Anemometry/Anemometry Sub Vis/LDA/Beam_Check_Positions.vi") -> (appended path=w247:path)
            n191 = Open VI Reference(type specifier VI Refnum (for type only)=refnum<vi> refnum, vi path=w247) -> (vi reference=w249:refnum<vi>, error out=w250:errorcluster)  [unwired: 1 in, 3 out]
            n192 = property class="VI Interface Type 3"(reference=w249, error in=w250, "Front Panel Window:Open"=TRUE) -> (reference out=w252:refnum<vi>, error out=w253:errorcluster)
            n193 = call-by-ref "?"(reference=w252, error in=w253, "Mode"=T41."Load From Excel File") -> (reference out=w254:refnum<vi>, error out=w255:errorcluster)  [unwired: 2 in, 1 out]
            n194 = Close Reference(reference=w254, error in (no error)=w255) -> ()  [unwired: 1 out]
          }
          event Mouse Down? {
            n195 = event-data() -> ()  [unwired: 5 out]
            n196 = global read "Constants_global.vi" "EnFlo SW Folder"() -> (w258:path)
            n197 = Build Path(base path=w258, name or relative path=path "Anemometry/Utilities/Hydrosonic_Manual.vi") -> (appended path=w261:path)
            n198 = call "Open_Close_Front_Panel.ph.vi"("Front Panel Window:Open"=TRUE, "VI path"=w261) -> ()  [unwired: 2 out]
            n199 = event-data() -> ()  [unwired: 1 in, 5 out]
          }
          event "Top Level Traverse": Mouse Down {
            n200 = event-data() -> ()  [unwired: 9 out]
            n201 = global read "Constants_global.vi" "EnFlo SW Folder"() -> (w262:path)
            n202 = Build Path(base path=w262, name or relative path=path "Anemometry/Utilities/Top_Level_Move_Traverse.vi") -> (appended path=w265:path)
            n203 = call "Open_Close_Front_Panel.ph.vi"("Front Panel Window:Open"=TRUE, "VI path"=w265) -> ()  [unwired: 2 out]
          }
          event "Post_Pro_Results_Hierarchy": Mouse Down {
            n204 = event-data() -> ()  [unwired: 9 out]
            n205 = global read "Constants_global.vi" "EnFlo SW Folder"() -> (w266:path)
            n206 = Build Path(base path=w266, name or relative path=path "Anemometry/Utilities/Post_Pro_Results_Hierarchy.vi") -> (appended path=w269:path)
            n207 = call "Open_Close_Front_Panel.ph.vi"("Front Panel Window:Open"=TRUE, "VI path"=w269) -> ()  [unwired: 2 out]
          }
          event Mouse Down? {
            n208 = event-data() -> ()  [unwired: 5 out]
            n209 = global read "Constants_global.vi" "EnFlo SW Folder"() -> (w270:path)
            n210 = Build Path(base path=w270, name or relative path=path "ADAM Client/ADAM client VIs/Fast_FID_Valve_Control.vi") -> (appended path=w273:path)
            n211 = call "Open_Close_Front_Panel.ph.vi"("Front Panel Window:Open"=TRUE, "VI path"=w273) -> ()  [unwired: 2 out]
            n212 = event-data() -> ()  [unwired: 1 in, 5 out]
          }
          event Mouse Down? {
            n213 = event-data() -> ()  [unwired: 5 out]
            n214 = global read "Constants_global.vi" "EnFlo SW Folder"() -> (w274:path)
            n215 = Build Path(base path=w274, name or relative path=path "Anemometry/Utilities/Preference_Panel.vi") -> (appended path=w283:path)
            n216 = Open VI Reference(type specifier VI Refnum (for type only)=refnum<vi> refnum, vi path=w283) -> (vi reference=w276:refnum<vi>, error out=w277:errorcluster)  [unwired: 1 in, 3 out]
            n217 = property class="VI Interface Type 4"(reference=w276, error in=w277, "Front Panel Window:Open"=TRUE) -> (reference out=w279:refnum<vi>, error out=w280:errorcluster)
            n218 = call-by-ref "?"(reference=w279, error in=w280, "Mode"=Preference_Mode."Load, Edit then Save") -> (reference out=w281:refnum<vi>, error out=w282:errorcluster)
            n219 = Close Reference(reference=w281, error in (no error)=w282) -> ()  [unwired: 1 out]
            n220 = event-data("Discard?"=TRUE) -> ()  [unwired: 1 in, 4 out]
          }
          event Mouse Down? {
            n221 = event-data() -> ()  [unwired: 5 out]
            n222 = global read "Constants_global.vi" "EnFlo SW Folder"() -> (w290:path)
            n223 = Build Path(base path=w290, name or relative path=path "ADAM Client/Sub VIs/Gas_Setup.vi") -> (appended path=w297:path)
            n224 = Open VI Reference(type specifier VI Refnum (for type only)=refnum<vi> refnum, vi path=w297) -> (vi reference=w293:refnum<vi>, error out=w294:errorcluster)  [unwired: 1 in, 3 out]
            n225 = property class="VI Interface Type 5"(reference=w293, error in=w294, "Front Panel Window:Open"=TRUE) -> (reference out=w298:refnum<vi>, error out=w296:errorcluster)
            n226 = call-by-ref "?"(reference=w298, error in=w296) -> (reference out=w288:refnum<vi>, error out=w287:errorcluster)  [unwired: 9 in]
            n227 = Close Reference(reference=w288, error in (no error)=w287) -> ()  [unwired: 1 out]
            n228 = event-data("Discard?"=TRUE) -> ()  [unwired: 1 in, 4 out]
          }
          event Mouse Down? {
            n229 = event-data() -> ()  [unwired: 5 out]
            n230 = global read "Constants_global.vi" "EnFlo SW Folder"() -> (w302:path)
            n231 = Build Path(base path=w302, name or relative path=path "ADAM Client/Sub VIs/User_Metadata.vi") -> (appended path=w309:path)
            n232 = Open VI Reference(type specifier VI Refnum (for type only)=refnum<vi> refnum, vi path=w309) -> (vi reference=w305:refnum<vi>, error out=w306:errorcluster)  [unwired: 1 in, 3 out]
            n233 = property class="VI Interface Type 5"(reference=w305, error in=w306, "Front Panel Window:Open"=TRUE) -> (reference out=w310:refnum<vi>, error out=w308:errorcluster)
            n234 = call-by-ref "?"(reference=w310, error in=w308) -> (reference out=w300:refnum<vi>, error out=w299:errorcluster)  [unwired: 9 in]
            n235 = Close Reference(reference=w300, error in (no error)=w299) -> ()  [unwired: 1 out]
            n236 = event-data("Discard?"=TRUE) -> ()  [unwired: 1 in, 4 out]
          }
          event Mouse Down? {
            n237 = event-data() -> ()  [unwired: 5 out]
            n238 = global read "Constants_global.vi" "EnFlo SW Folder"() -> (w316:path)
            n239 = Build Path(base path=w316, name or relative path=path "ADAM Client/Sub VIs/EnFlo_Tunnel_Setup.vi") -> (appended path=w319:path)
            n240 = Open VI Reference(type specifier VI Refnum (for type only)=refnum<vi> refnum, vi path=w319) -> (vi reference=w313:refnum<vi>, error out=w312:errorcluster)  [unwired: 1 in, 3 out]
            n241 = call-by-ref "?"(reference=w313, error in=w312) -> (reference out=w315:refnum<vi>, error out=w314:errorcluster)  [unwired: 9 in]
            n242 = Close Reference(reference=w315, error in (no error)=w314) -> ()  [unwired: 1 out]
            n243 = event-data("Discard?"=TRUE) -> ()  [unwired: 1 in, 4 out]
          }
          event Mouse Down? {
            w330 = TRUE  # Show Panel?
            n244 = event-data() -> ()  [unwired: 5 out]
            n245 = global read "Constants_global.vi" "EnFlo SW Folder"() -> (w325:path)
            n246 = Build Path(base path=w325, name or relative path=path "Anemometry/Anemometry Sub Vis/Gen Trav/Traverse_Space.vi") -> (appended path=w328:path)
            n247 = global read "Trav_pos_global.vi" "Default Traverse Setup"() -> (w320:string)
            n248 = Open VI Reference(type specifier VI Refnum (for type only)=refnum<vi> refnum, vi path=w328) -> (vi reference=w329:refnum<vi>, error out=w321:errorcluster)  [unwired: 1 in, 3 out]
            n249 = call-by-ref "?"(reference=w329, error in=w321, "Show Panel?"=w330, "Traverse Setup"=w320) -> (reference out=w323:refnum<vi>, error out=w322:errorcluster)  [unwired: 8 in, 1 out]
            n250 = Close Reference(reference=w323, error in (no error)=w322) -> ()  [unwired: 1 out]
            n251 = event-data("Discard?"=TRUE) -> ()  [unwired: 1 in, 4 out]
          }
          event Mouse Down? {
            n252 = event-data() -> ()  [unwired: 5 out]
            n253 = global read "Constants_global.vi" "EnFlo SW Folder"() -> (w332:path)
            n254 = Build Path(base path=w332, name or relative path=path "Anemometry/Anemometry Sub Vis/Traverse vi's/EnFlo Tunnel specific/Check_EnFlo_Arm.vi") -> (appended path=w334:path)
            n255 = call "Open_Close_Front_Panel.ph.vi"("Front Panel Window:Open"=TRUE, "VI path"=w334) -> ()  [unwired: 2 out]
            n256 = event-data() -> ()  [unwired: 1 in, 2 out]
          }
          event Mouse Down? {
            n257 = event-data() -> ()  [unwired: 5 out]
            n258 = global read "Constants_global.vi" "EnFlo SW Folder"() -> (w342:path)
            n259 = Build Path(base path=w342, name or relative path=path "Anemometry/Anemometry Sub Vis/Gen Trav/3D_Traverse_move.vi") -> (appended path=w339:path)
            n260 = Strip Path(path=w339) -> (name=w338:string)  [unwired: 1 out]
            n261 = Open VI Reference(vi path=w338) -> (vi reference=w340:refnum<vi>, error out=w341:errorcluster)  [unwired: 1 in, 4 out]
            n262 = property class="VI"(reference=w340, error in=w341) -> (reference out=w336:refnum<vi>, error out=w335:errorcluster, "Front Panel Window:Open"=w337:bool)
            n263 = case shown="False" w337 {
              tunnel: w339 -> [w344 _]
              tunnel: w336 -> [_ w361]
              tunnel: w335 -> [_ w360]
              frame False {
                n264 = global read "Trav_pos_global.vi" "Work in Tunnel Coordinates?"() -> (w354:T48)
                n265 = global read "Trav_pos_global.vi" "Default Traverse Setup"() -> (w352:string)
                n266 = Open VI Reference(type specifier VI Refnum (for type only)=refnum<vi> refnum, vi path=w344) -> (vi reference=w348:refnum<vi>, error out=w349:errorcluster)  [unwired: 1 in, 3 out]
                n267 = property class="VI Interface Type 6"(reference=w348, error in=w349, "Front Panel Window:Open"=TRUE) -> (reference out=w345:refnum<vi>, error out=w346:errorcluster)
                n268 = call-by-ref "?"(reference=w345, error in=w346, "Mode"=Trav_mode."Read traverse position", "Work in Tunnel Coordinates"=w354, "Simulate/Run"=User_Specific_mode."Run VI", "Traverse name"=w352) -> (reference out=w350:refnum<vi>, error out=w351:errorcluster)  [unwired: 9 in, 3 out]
                n269 = Close Reference(reference=w350, error in (no error)=w351) -> ()  [unwired: 1 out]
              }
              frame True {
                n270 = property class="VI"(reference=w361, error in=w360, "Front Panel Window:Open"=TRUE) -> (reference out=w359:refnum<vi>, error out=w358:errorcluster)
                n271 = Close Reference(reference=w359, error in (no error)=w358) -> ()  [unwired: 1 out]
              }
            }
            n272 = event-data() -> ()  [unwired: 1 in, 5 out]
          }
          event Mouse Down? {
            n273 = event-data() -> ()  [unwired: 5 out]
            n274 = Open VI Reference(vi path="Multi_Run_Prog.vi") -> (vi reference=w367:refnum<vi>, error out=w366:errorcluster)  [unwired: 1 in, 4 out]
            n275 = property class="VI"(reference=w367, error in=w366, "Front Panel Window:Open"=TRUE) -> (reference out=w364:refnum<vi>, error out=w365:errorcluster)
            n276 = Close Reference(reference=w364, error in (no error)=w365) -> (error out=w362:errorcluster)
            n277 = Unbundle By Name(w362) -> ("status"=w369:bool)
            n278 = case shown="True" w369 {
              frame False {
              }
              frame True {
                n279 = global read "Constants_global.vi" "EnFlo SW Folder"() -> (w377:path)
                n280 = call "Setup_Filepath.vi"("Setup File Type"=Setup_Filetype."General", "Filename in"="Multi_Run_Filename.txt" ("name or relative path")) -> ("Filename Out"=w370:path)  [unwired: 1 out]
                n281 = Build Path(base path=w377, name or relative path=path "Anemometry/Multi_Run_Prog.vi") -> (appended path=w376:path)
                n282 = call "Read_File_Simple.vi"("Filename"=w370) -> ("string"=w375:string)  [unwired: 2 in, 7 out]
                n283 = String To Path(string=w375) -> (path=w373:path)
                n284 = call "Does_file_exist_(simple).vi"("Pathname"=w373) -> ("exists?"=w374:bool)
                n285 = case shown="False" w374 {
                  tunnel: w376 -> [w379 w391]
                  tunnel: w373 -> [_ w388]
                  frame False {
                    n286 = call "Open_Close_Front_Panel.ph.vi"("Front Panel Window:Open"=TRUE, "VI path"=w379) -> ()  [unwired: 2 out]
                  }
                  frame True {
                    n287 = Open VI Reference(type specifier VI Refnum (for type only)=refnum<vi> refnum, vi path=w391) -> (vi reference=w387:refnum<vi>, error out=w386:errorcluster)  [unwired: 1 in, 3 out]
                    n288 = property class="VI Interface Type 7"(reference=w387, error in=w386, "Front Panel Window:Open"=TRUE) -> (reference out=w384:refnum<vi>, error out=w385:errorcluster)
                    n289 = call-by-ref "?"(reference=w384, error in=w385, "Command filename"=w388, "Setup mode"=T46."Load Command File") -> (reference out=w383:refnum<vi>, error out=w382:errorcluster)  [unwired: 18 in]
                    n290 = Close Reference(reference=w383, error in (no error)=w382) -> ()  [unwired: 1 out]
                  }
                }
              }
            }
            n291 = event-data() -> ()  [unwired: 1 in, 5 out]
          }
          event Mouse Down? {
            w393 = "Calibration.vi" ("name or relative path")
            n292 = event-data() -> ()  [unwired: 5 out]
            n293 = global read "Constants_global.vi" "EnFlo SW Folder"() -> (w399:path)
            n294 = Open VI Reference(vi path=w393) -> (vi reference=w397:refnum<vi>, error out=w396:errorcluster)  [unwired: 1 in, 4 out]
            n295 = Build Path(base path=w399, name or relative path="Anemometry") -> (appended path=w402:path)
            n296 = property class="VI"(reference=w397, error in=w396, "Front Panel Window:Open"=TRUE) -> (reference out=w394:refnum<vi>, error out=w395:errorcluster)
            n297 = Build Path(base path=w402, name or relative path=w393) -> (appended path=w400:path)
            n298 = Close Reference(reference=w394, error in (no error)=w395) -> (error out=w392:errorcluster)
            n299 = Unbundle By Name(w392) -> ("status"=w401:bool)
            n300 = case shown="True" w401 {
              tunnel: w400 -> [_ w404]
              tunnel: w392 -> [_ _]
              frame False {
              }
              frame True {
                n301 = stacked-sequence {
                  seq-local: [w410 _] -> [_ w417]
                  tunnel: w404 -> [_ w418]
                  frame #0 {
                    n302 = call "Setup_Filepath.vi"("Setup File Type"=Setup_Filetype."Calibration Setups", "Filename in"="Current_Setup.xls") -> ("Filename Out"=w405:path)  [unwired: 1 out]
                    n303 = call "Read_File_Simple.vi"("Filename"=w405) -> ("string"=w414:string)  [unwired: 2 in, 7 out]
                    n304 = Format Into String(format string="Calibration Setup File   %s", w405) -> (resulting string=w408:string)  [unwired: 2 in, 1 out]
                    n305 = call "Get_string_subset.vi"("String Name"=w408, "String to split"=w414, "File Label"="Raw data header") -> ("Output string"=w412:string)  [unwired: 1 in, 1 out]
                    n306 = call "Get_Characters_from_string.vi"("Input string"=w412, "Variable name"="Calib filename") -> ("Value"=w411:string)  [unwired: 1 in, 1 out]
                    n307 = call "String_to_Pathname.vi"("Input String"=w411) -> ("path"=w410:path)
                  }
                  frame #1 {
                    n308 = call "Does_file_exist_(simple).vi"("Pathname"=w417) -> ("exists?"=w416:bool)
                    n309 = case shown="True" w416 {
                      tunnel: w418 -> [w419 w434]
                      tunnel: w417 -> [_ w428]
                      frame False {
                        n310 = call "Open_Close_Front_Panel.ph.vi"("Front Panel Window:Open"=TRUE, "VI path"=w419) -> ()  [unwired: 2 out]
                      }
                      frame True {
                        w426 = TRUE ("Front Panel Window:Open")
                        n311 = Open VI Reference(type specifier VI Refnum (for type only)=refnum<vi> refnum, vi path=w434) -> (vi reference=w432:refnum<vi>, error out=w427:errorcluster)  [unwired: 1 in, 3 out]
                        n312 = property class="VI Interface Type 8"(reference=w432, error in=w427, "Front Panel Window:Open"=w426, "Front Panel Window:Auto Center (Deprecated)"=w426) -> (reference out=w431:refnum<vi>, error out=w430:errorcluster)
                        n313 = call-by-ref "?"(reference=w431, error in=w430, "Mode"=Calib_mode."Setup Front Panel", "Calib file"=w428) -> (reference out=w424:refnum<vi>, error out=w423:errorcluster)  [unwired: 15 in, 3 out]
                        n314 = property class="VI Interface Type 8"(reference=w424, error in=w423, "Front Panel Window:Auto Center (Deprecated)"=FALSE ("Front Panel Window:Auto Center")) -> (reference out=w422:refnum<vi>, error out=w421:errorcluster)
                        n315 = Close Reference(reference=w422, error in (no error)=w421) -> ()  [unwired: 1 out]
                      }
                    }
                  }
                }
              }
            }
            n316 = event-data() -> ()  [unwired: 1 in, 5 out]
          }
          event "stop": Mouse Down? {
            n317 = event-data() -> ()  [unwired: 5 out]
            n318 = flat-sequence {
              frame #0 {
                n319 = global write "Dynamic_call_global.ph.vi" "EnFlo Hub running?"(FALSE ("EnFlo Hub running?")) -> ()
              }
              frame #1 {
                n320 = Stop(stop? (T)=TRUE) -> ()
              }
            }
            n321 = event-data() -> ()  [unwired: 1 in, 4 out]
          }
          event "Rig_Control": Value Change {
            n322 = event-data() -> ("OldVal"=w438:cluster{"Ch Name":string, "Boolean":bool}[], "NewVal"=w437:cluster{"Ch Name":string, "Boolean":bool}[])  [unwired: 5 out]
            n323 = for {
              tunnel: w438 -> [w444] mode=indexing
              tunnel: w437 -> [w443] mode=indexing
              n324 = Unbundle By Name(w444) -> ("Ch Name"=w441:string, "Boolean"=w442:bool)
              n325 = Unbundle By Name(w443) -> ("Boolean"=w440:bool)  [unwired: 1 out]
              n326 = Not Equal?(x=w442, y=w440) -> (x != y?=w439:bool)
              n327 = case shown="True" w439 {
                tunnel: w441 -> [_ w446]
                tunnel: w440 -> [_ w453]
                frame False {
                }
                frame True {
                  n328 = Select(t="TRUE", s=w453, f="FALSE") -> (s? t:f=w445:string)
                  n329 = Select(t=1.0, s=w453, f=0.0) -> (s? t:f=w452:dbl)
                  n330 = Format Into String(format string="Are you sure you want to make %s %s?", w446, w445) -> (resulting string=w455:string)  [unwired: 2 in, 1 out]
                  n331 = Format Into String(format string="Make  %s  %s", w446, w445) -> (resulting string=w447:string)  [unwired: 2 in, 1 out]
                  n332 = Two Button Dialog(message=w455, 1:w447, 2:"Cancel" ("T button name (\"OK\")")) -> (T button?=w449:bool)
                  n333 = case shown="False" w449 {
                    tunnel: w446 -> [w460 _]
                    tunnel: w452 -> [w459 _]
                    frame False {
                      n334 = Build Array(w459) -> (w462:dbl[])
                      n335 = Build Array(w460) -> (w461:string[])
                      n336 = call "ASYNC_Adam_client.vi"("Values"=w462, "Channel Names"=w461) -> ()  [unwired: 1 in, 2 out]
                    }
                    frame True {
                    }
                  }
                }
              }
            }
          }
        }
      }
    }
    "Numeric" <- w8
  }
  n337 = while {
    shift-left: _ -> [w467]
    shift-right: [w468] -> _
    shift-left: "Initialise" -> [w466]
    shift-right: [w469] -> _
    tunnel: "ADAM_Chs_to_Enable.txt" ("name or relative path") -> [w464]
    tunnel: "ADAM_Chs_to_View.txt" ("name or relative path") -> [w463]
    i -> [w465]
    stop <- TRUE continue-if-true
    n338 = case shown="\"Initialise\"" w466 {
      tunnel: ["End" "Initialise" "Wait for call remote sub vi occurrence" "Check type of VI to launch" w539 "Wait until remote sub vi is opened" "Update opened vis array" "Update opened vis array" "Update opened vis array" "Wait until remote sub vi is opened" "Wait for call remote sub vi occurrence"] -> w469
      tunnel: [w471 w484 w489 errorcluster {"status"=FALSE, "code"=0, "source"=""} ("error out") w535 w550 w580 w597 w612 w652 w672] -> w468
      tunnel: w467 -> [w471 w484 w489 _ w535 w550 _ _ _ w652 w672]
      tunnel: w466 -> [w473 _ _ _ _ _ _ _ _ _ _]
      tunnel: w465 -> [_ _ _ _ _ _ _ _ _ _ _]
      tunnel: w464 -> [_ _ w486 _ _ _ _ _ _ _ _]
      tunnel: w463 -> [_ _ w485 _ _ _ _ _ _ _ _]
      frame "No match", Default {
        n339 = Current VI's Path() -> (path=w474:path)
        n340 = Format Into String(format string="The Case\"%s\" was not Matched\nin VI named\n'%s\"" ("Format String"), w473, w474) -> (resulting string=w477:string)  [unwired: 2 in, 1 out]
        n341 = One Button Dialog(message=w477, button name ("OK")="STOP") -> (true=w475:bool)
        n342 = Stop(stop? (T)=w475) -> ()
      }
      frame "Never run" {
        # "These globals are here to make sure they stay in momory\nafter \"Preference Panel\" has finished running"
        n343 = call "Email_With_Log.vi"() -> ()  [unwired: 4 in, 3 out]
        n344 = call "Remember_value.vi"() -> ()  [unwired: 3 in, 1 out]
        n345 = call "Output_Trav_Pos.vi"() -> ()  [unwired: 5 in, 1 out]
        n346 = call "Read_Write_Local_table.vi"() -> ()  [unwired: 3 in, 3 out]
        n347 = call "Overhead_Factor.vi"() -> ()  [unwired: 4 in, 1 out]
        n348 = global read "Trav_pos_global.vi" "Dummy Measurement?"() -> (→"Dummy Measurement":bool)
        n349 = global read "PWAtasksGLOBAL.vi" "Analogue Dev Name"() -> (→"Analogue Dev Name":string)
        n350 = global read "Constants_global.vi" "All_Users"() -> (→"All Users":path)
        n351 = global read "Preference_global.vi" "Rig Setup"() -> (→"Rig Name":string)
      }
      frame "Initialise" {
        n352 = stacked-sequence {
          tunnel: w486 -> [_ _ _ _ w527]
          tunnel: w485 -> [_ _ _ _ w523]
          frame #0 {
            n353 = Generate Occurrence() -> (w510:refnum<k4>)
            n354 = global write "Dynamic_call_global.ph.vi" "Call Remote Subvi"(w510) -> ()
            n355 = Generate Occurrence() -> (w509:refnum<k4>)
            n356 = global write "Dynamic_call_global.ph.vi" "Remote Subvi Opened"(w509) -> ()
            n357 = Initialize Array("", 0) -> (w507:string[])
            n358 = global write "Dynamic_call_global.ph.vi" "Opened VIs"(w507) -> ()
            n359 = global write "Email_transfer_global.vi" "Busy?"(FALSE ("Busy?")) -> ()
            n360 = Current VI's Path() -> (path=w499:path)
            n361 = Strip Path(path=w499) -> (stripped path=w497:path)  [unwired: 1 out]
            n362 = Build Path(base path=w497, name or relative path="Utilities") -> (appended path=w495:path)
            n363 = Build Path(base path=w495, name or relative path="Preference_Panel.vi") -> (appended path=w494:path)
            n364 = Get Date/Time In Seconds() -> (seconds since 1Jan1904=w505:timestamp)
            n365 = To Double Precision Float(number=w505) -> (double precision float=w504:dbl)
            n366 = Open VI Reference(type specifier VI Refnum (for type only)=refnum<vi> refnum, vi path=w494) -> (vi reference=w500:refnum<vi>, error out=w501:errorcluster)  [unwired: 1 in, 3 out]
            n367 = global write "Meas_global.vi" "Start Time of experiment"(w504) -> ()
            n368 = global write "Meas_global.vi" "Post Process"(Post_Process."Post Process Raw Data File" ("Post Process")) -> ()
            n369 = call-by-ref "?"(reference=w500, error in=w501, "Mode"=Preference_Mode."Load Preferences from file") -> (reference out=w502:refnum<vi>, error out=w503:errorcluster)
            n370 = Close Reference(reference=w502, error in (no error)=w503) -> ()  [unwired: 1 out]
          }
          frame #1 {
            w511 = TRUE  # OK
            n371 = call "Get_users_email_addresses.vi"("OK"=w511) -> ()  [unwired: 5 out]
          }
          frame #2 {
            n372 = Current VI's Path() -> (path=w520:path)
            n373 = Open VI Reference(vi path=w520) -> (vi reference=w519:refnum<vi>, error out=w518:errorcluster)  [unwired: 1 in, 4 out]
            n374 = call "Last_modified_date.vi"("Update Now"=TRUE) -> ("RevisionString"=w512:string)  [unwired: 1 out]
            n375 = property class="VI"(reference=w519, error in=w518, "Front Panel Window:Open"=TRUE, "Front Panel Window:Is Frontmost"=FALSE) -> (reference out=w517:refnum<vi>, error out=w516:errorcluster)
            n376 = global write "Meas_global.vi" "ProgRevisionInfo"(w512) -> ()
            n377 = Close Reference(reference=w517, error in (no error)=w516) -> ()  [unwired: 1 out]
          }
          frame #3 {
            n378 = global write "Dynamic_call_global.ph.vi" "EnFlo Hub running?"(TRUE ("EnFlo Hub running?")) -> ()
          }
          frame #4 {
            n379 = global read "Constants_global.vi" "All_Users"() -> (w524:path)
            n380 = Build Path(base path=w524, name or relative path=w523) -> (appended path=w526:path)
            n381 = Build Path(base path=w524, name or relative path=w527) -> (appended path=w529:path)
            n382 = call "Read_File_Simple.vi"("Filename"=w526) -> ("string"=w525:string)  [unwired: 2 in, 7 out]
            n383 = call "Read_File_Simple.vi"("Filename"=w529) -> ("string"=w530:string)  [unwired: 2 in, 7 out]
            n384 = call "Get_array_values_fr_String.vi"("String Value"=w525) -> ("String array"=→"List of ADAM channels to view":string[])  [unwired: 1 out]
            n385 = call "Get_array_values_fr_String.vi"("String Value"=w530) -> ("String array"=→"List of ADAM control channels":string[])  [unwired: 1 out]
          }
        }
        "Iterations" <- 0 ("Iterations")
      }
      frame "Wait for call remote sub vi occurrence" {
        n386 = global read "Dynamic_call_global.ph.vi" "Call Remote Subvi"() -> (w533:refnum<k4>)
        n387 = Wait on Occurrence(2:w533) -> ()  [unwired: 3 out]
      }
      frame "Check type of VI to launch" {
        n388 = global read "Dynamic_call_global.ph.vi" "VI name to launch"() -> (w537:string)
        n389 = Match Pattern(string=w537, regular expression=";") -> (before substring=w534:string, after substring=w536:string)  [unwired: 3 out]
        n390 = case shown="\"Open LDA PWA & An\"" w534 {
          tunnel: ["Open vi" "Open application reference" "Open Analogue input server" w547] -> w539
          tunnel: [w542 w544 w546 w548] -> w538
          tunnel: w537 -> [w542 _ _ _]
          tunnel: w536 -> [_ w544 w546 w548]
          tunnel: w534 -> [_ _ _ w547]
          frame "Other", Default {
          }
          frame "Open Application Reference" {
          }
          frame "Open Analogue Input VI" {
          }
          frame "Open LDA PWA & An" {
          }
        }
        "VI Name" <- w538
      }
      frame "Open application reference" {
        n391 = local read "VI Name"() -> (w551:string)
        n392 = Match Pattern(string=w551, regular expression=";") -> (before substring=w559:string, after substring=w560:string)  [unwired: 3 out]
        n393 = Decimal String To Number(string=w560) -> (number=w561:i32)  [unwired: 3 out]
        n394 = To Unsigned Long Integer(number=w561) -> (unsigned 32bit integer=w558:u32)
        n395 = call "App_Ref_Global.vi"("Mode"=App_Global."Read Global") -> ("Output Array"=w557:T50[])  [unwired: 1 in, 1 out]
        n396 = Open Application Reference(10:w558, 11:w559) -> (0:w552:errorcluster, 3:w556:refnum<vi>)  [unwired: 1 in, 1 out]
        n397 = for {
          tunnel: w557 -> [w563] mode=indexing
          tunnel: w551 -> [w567]
          tunnel: w556 -> [w565]
          tunnel: [w564] -> w555 mode=indexing
          n398 = Unbundle By Name(w563) -> ("Server IP & Port No"=w568:string)
          n399 = Equal?(x=w568, y=w567) -> (x = y?=w566:bool)
          n400 = case shown="False" w566 {
            tunnel: w565 -> [_ w572]
            tunnel: [w569 w571] -> w564
            tunnel: w563 -> [w569 w570]
            frame False {
            }
            frame True {
              n401 = Bundle By Name(cluster=w570, "Application reference"=w572) -> (w571:T50)
            }
          }
        }
        n402 = global write "Dynamic_call_global.ph.vi" "Error Cluster"(w552) -> ()
        n403 = call "App_Ref_Global.vi"("Input Array"=w555, "Mode"=App_Global."Write to Global") -> ()  [unwired: 2 out]
      }
      frame "Open Analogue input server" {
        n404 = local read "VI Name"() -> (w577:string)
        n405 = call "Get_link_info.vi"("VI Name"=w577) -> ("Path name"=w574:path, "Application reference"=w575:refnum<vi>, "Local Call?"=w576:bool)  [unwired: 1 out]
        n406 = global read "Dynamic_call_global.ph.vi" "Analogue Input"() -> (w579:refnum<vi>)
        n407 = case shown="True" w576 {
          tunnel: w579 -> [w585 w589]
          tunnel: [w581 w588] -> w578
          tunnel: [w584 w587] -> w580
          tunnel: w577 -> [w583 _]
          tunnel: w575 -> [w582 _]
          tunnel: w574 -> [_ w586]
          frame False {
            n408 = Open VI Reference(type specifier VI Refnum (for type only)=w585, application reference (local)=w582, vi path=w583) -> (vi reference=w581:refnum<vi>, error out=w584:errorcluster)  [unwired: 1 in, 2 out]
          }
          frame True {
            n409 = Open VI Reference(type specifier VI Refnum (for type only)=w589, vi path=w586) -> (vi reference=w588:refnum<vi>, error out=w587:errorcluster)  [unwired: 1 in, 3 out]
          }
        }
        n410 = global write "Dynamic_call_global.ph.vi" "Analogue Input"(w578) -> ()
      }
      frame "Open LDA PWA & An" {
        n411 = local read "VI Name"() -> (w594:string)
        n412 = call "Get_link_info.vi"("VI Name"=w594) -> ("Path name"=w591:path, "Application reference"=w592:refnum<vi>, "Local Call?"=w593:bool)  [unwired: 1 out]
        n413 = global read "Dynamic_call_global.ph.vi" "Take LDA PWA & An"() -> (w596:refnum<vi>)
        n414 = case shown="True" w593 {
          tunnel: w596 -> [w602 w606]
          tunnel: [w598 w605] -> w595
          tunnel: [w601 w604] -> w597
          tunnel: w594 -> [w600 _]
          tunnel: w592 -> [w599 _]
          tunnel: w591 -> [_ w603]
          frame False {
            n415 = Open VI Reference(type specifier VI Refnum (for type only)=w602, application reference (local)=w599, vi path=w600) -> (vi reference=w598:refnum<vi>, error out=w601:errorcluster)  [unwired: 1 in, 2 out]
          }
          frame True {
            n416 = Open VI Reference(type specifier VI Refnum (for type only)=w606, vi path=w603) -> (vi reference=w605:refnum<vi>, error out=w604:errorcluster)  [unwired: 1 in, 3 out]
          }
        }
        n417 = global write "Dynamic_call_global.ph.vi" "Take LDA PWA & An"(w595) -> ()
      }
      frame "Open vi" {
        n418 = local read "VI Name"() -> (w611:string)
        n419 = call "Get_link_info.vi"("VI Name"=w611) -> ("Path name"=w610:path, "Application reference"=w609:refnum<vi>, "Local Call?"=w608:bool)  [unwired: 1 out]
        n420 = case shown="\"No Match\", Default" w611 {
          tunnel: [w613 w622 w634] -> w612
          tunnel: w611 -> [w618 w621 w638]
          tunnel: w610 -> [_ _ w635]
          tunnel: w609 -> [_ w620 w637]
          tunnel: w608 -> [_ w619 w636]
          frame "No Match", Default {
            n421 = Format Into String(format string="VI named \"%s\" Not matched" ("Format String"), w618) -> (resulting string=w615:string)  [unwired: 2 in, 1 out]
            n422 = Bundle By Name(cluster=errorcluster {"status"=FALSE, "code"=0, "source"=""} ("error out"), "source"=w615, "status"=TRUE ("Bundle Element")) -> (w613:errorcluster)
          }
          frame "Program_Active_server.vi" {
            n423 = global read "Dynamic_call_global.ph.vi" "Program Active server"() -> (w624:refnum<vi>)
            n424 = case shown="True" w619 {
              tunnel: w624 -> [w629 w633]
              tunnel: [w628 w632] -> w623
              tunnel: [w627 w631] -> w622
              tunnel: w621 -> [w626 w630]
              tunnel: w620 -> [w625 _]
              frame False {
                n425 = Open VI Reference(type specifier VI Refnum (for type only)=w629, application reference (local)=w625, vi path=w626) -> (vi reference=w628:refnum<vi>, error out=w627:errorcluster)  [unwired: 1 in, 2 out]
              }
              frame True {
                n426 = Open VI Reference(type specifier VI Refnum (for type only)=w633, vi path=w630) -> (vi reference=w632:refnum<vi>, error out=w631:errorcluster)  [unwired: 1 in, 3 out]
              }
            }
            n427 = global write "Dynamic_call_global.ph.vi" "Program Active server"(w623) -> ()
          }
          frame "GPIB_Server.vi" {
            n428 = global read "Dynamic_call_global.ph.vi" "GPIB_Server.vi"() -> (w640:refnum<vi>)
            n429 = case shown="False" w636 {
              tunnel: w640 -> [w645 w649]
              tunnel: [w644 w648] -> w639
              tunnel: [w643 w647] -> w634
              tunnel: w638 -> [w641 _]
              tunnel: w637 -> [w642 _]
              tunnel: w635 -> [_ w646]
              frame False {
                n430 = Open VI Reference(type specifier VI Refnum (for type only)=w645, application reference (local)=w642, vi path=w641) -> (vi reference=w644:refnum<vi>, error out=w643:errorcluster)  [unwired: 1 in, 2 out]
              }
              frame True {
                n431 = Open VI Reference(type specifier VI Refnum (for type only)=w649, vi path=w646) -> (vi reference=w648:refnum<vi>, error out=w647:errorcluster)  [unwired: 1 in, 3 out]
              }
            }
            n432 = global write "Dynamic_call_global.ph.vi" "GPIB_Server.vi"(w639) -> ()
          }
        }
      }
      frame "Update opened vis array" {
        w654 = TRUE  # Dialog Box
        n433 = local read "VI Name"() -> (w653:string)
        n434 = Unbundle By Name(w652) -> ("status"=w657:bool, "source"=w655:string)
        n435 = case shown="True" w657 {
          tunnel: w652 -> [w659 w668]
          tunnel: [w659 w667] -> w656
          tunnel: w653 -> [w660 w663]
          tunnel: w655 -> [_ w666]
          frame False {
            n436 = global read "Dynamic_call_global.ph.vi" "Opened VIs"() -> (w661:string[])
            n437 = To Upper Case(1:w660) -> (0:w658:string)
            n438 = Build Array (concatenate)(w661, w658) -> (w662:string[])
            n439 = global write "Dynamic_call_global.ph.vi" "Opened VIs"(w662) -> ()
          }
          frame True {
            n440 = Concatenate Strings(w663, " " ("Substring"), w666) -> (w664:string)
            n441 = Bundle By Name(cluster=w668, "source"=w664) -> (w667:errorcluster)
          }
        }
        n442 = call "EnFlo_Error_Handler.vi"("error in (no error)"=w656, "Error Type"="Dynamic Call", "Dialog Box (T)"=w654) -> ()  [unwired: 3 out]
      }
      frame "Wait until remote sub vi is opened" {
        n443 = global read "Dynamic_call_global.ph.vi" "Remote Subvi Opened"() -> (w673:refnum<k4>)
        n444 = local read "Iterations"() -> (w671:i32)
        n445 = Increment(x=w671) -> (x+1=w670:i32)
        n446 = local write "Iterations"(w670) -> ()
        n447 = Set Occurrence(w673) -> ()
      }
    }
  }
  n448 = while {
    i -> [w674]
    stop <- FALSE stop-if-true
    n449 = stacked-sequence {
      tunnel: w674 -> [_ w722]
      frame #0 {
        n450 = global read "Dynamic_call_global.ph.vi" "EnFlo Hub running?"() -> (w678:bool)
        n451 = Equal?(x="Tab Control", y=T1."Adam Table" ("Tab Control")) -> (x = y?=w679:bool)
        n452 = And(x=w679, y=w678) -> (x .and. y?=w677:bool)
        n453 = case shown="True" w677 {
          frame True {
            n454 = local read "List of ADAM channels to view"() -> (w688:string[])
            n455 = local read "List of ADAM control channels"() -> (w691:string[])
            n456 = Build Array (concatenate)(w691, w688) -> (w690:string[])
            n457 = call "Get_Current_Scan_client.vi"("ADAM Ch Names"=w690) -> ("Ch Description Array"=w685:T52[], "Numerical Values"=w689:dbl[])  [unwired: 2 out]
            n458 = Array Size(array=w691) -> (size(s)=w686:i32)
            n459 = Array Subset(array=w685, index=w686) -> (w684:T52[])  [unwired: 1 in]
            n460 = Array Subset(array=w689, index=w686) -> (w683:dbl[])  [unwired: 1 in]
            n461 = for {
              tunnel: w684 -> [w698] mode=indexing
              tunnel: [w697] -> w682 mode=indexing
              tunnel: cluster{"Ch Name":string, "Numeric":dbl} {"Ch Name"="", "Numeric"=0.0} ("Cluster") -> [w696]
              tunnel: w683 -> [w694] mode=indexing
              n462 = Unbundle By Name(w698) -> ("Ch Name"=w695:string)
              n463 = Bundle By Name(cluster=w696, "Ch Name"=w695, "Numeric"=w694) -> (w697:cluster{"Ch Name":string, "Numeric":dbl})
            }
            "Current Values" <- w682
            n464 = for {
              N: w686 -> [_]
              tunnel: cluster{"Ch Name":string, "Boolean":bool} {"Ch Name"="", "Boolean"=FALSE} ("Cluster") -> [w705]
              tunnel: w685 -> [w704] mode=indexing
              tunnel: w689 -> [w702] mode=indexing
              tunnel: [w699] -> w692 mode=indexing
              n465 = Unbundle By Name(w704) -> ("Ch Name"=w703:string)
              n466 = Greater?(x=w702, y=0.5) -> (0:w700:bool)
              n467 = Bundle By Name(cluster=w705, "Ch Name"=w703, "Boolean"=w700) -> (w699:cluster{"Ch Name":string, "Boolean":bool})
            }
            n468 = local write "Rig_Control"(w692) -> ()
          }
          frame False {
          }
        }
      }
      frame #1 {
        w720 = 300 ("y")
        n469 = global read "Trav_pos_global.vi" "Sync to server now"() -> (w706:bool)
        n470 = Quotient & Remainder(x=w722, y=86400) -> (x-y*floor(x/y)=w723:i32)  [unwired: 1 out]
        n471 = Quotient & Remainder(x=w722, y=21600) -> (x-y*floor(x/y)=w719:i32)  [unwired: 1 out]
        n472 = Equal?(x=w723, y=w720) -> (x = y?=w717:bool)
        n473 = Equal?(x=w720, y=w719) -> (x = y?=w718:bool)
        n474 = Or(x=w717, y=w718) -> (x .or. y?=w710:bool)
        n475 = Select(t=3 ("Months of History to backup"), s=w717, f=1) -> (s? t:f=w714:i32)
        n476 = global read "Preference_global.vi" "Server Comms"() -> (w712:T51)
        n477 = Equal?(x=w712, y=Server_Comms."Server Link Healthy" ("Server Comms")) -> (x = y?=w711:bool)
        n478 = And(x=w710, y=w711) -> (x .and. y?=w708:bool)
        n479 = Compound Arithmetic op=OR(w706, "Sync to server now", w708) -> (w707:bool)
        n480 = case shown="True" w707 {
          tunnel: w714 -> [_ w725]
          frame False {
          }
          frame True {
            n481 = stacked-sequence {
              tunnel: w725 -> [w728 _]
              frame #0 {
                w726 = TRUE  # Check Updates on Server?
                w727 = TRUE  # Get all Server Files
                n482 = call "Backup_Client.vi"("Check Updates on Server?"=w726, "Get all Server Files"=w727, "Months of History to backup"=w728) -> ()  [unwired: 1 out]
              }
              frame #1 {
                w729 = FALSE ("Sync to server now")
                n483 = local write "Sync to server now"(w729) -> ()
                n484 = global write "Trav_pos_global.vi" "Sync to server now"(w729) -> ()
              }
            }
          }
        }
      }
    }
    n485 = Wait (ms)(milliseconds to wait=u32 1000) -> ()  [unwired: 1 out]
  }
